vi "Preference_Panel.vi"(0 "Mode":T1) -> ()   [LabVIEW 2010]
uses:
  Anemometry Sub Vis/Controls/Server_Comms.ctl
  Anemometry Sub Vis/Controls/Preference_Mode.ctl
  Anemometry Sub Vis/File/Setup_Filetype.ctl
  Anemometry Sub Vis/Controls/Overhead.ctl
  <vilib>/Instr/_visa.llb/VISA Find Search Mode.ctl
  ADAM Client/Sub VIs/ADAM Controls/Calib_type_ADAM.ctl
  ADAM Client/Sub VIs/ADAM Controls/Module_type_ADAM.ctl
  ADAM Client/Sub VIs/ADAM Controls/Ch_description_ADAM.ctl
  ADAM Client/Sub VIs/ADAM Controls/Function_ADAM.ctl
  ADAM Client/Sub VIs/ADAM Controls/Channel_State.ctl
  ADAM Client/Sub VIs/ADAM Controls/Address.ctl
  Anemometry Sub Vis/Globals/Constants_global.vi
  Anemometry Sub Vis/Globals/Preference_global.vi
  Anemometry Sub Vis/Globals/Trav_pos_global.vi
  Anemometry Sub Vis/Globals/Qnet_Globals.vi
  Anemometry Sub Vis/Acquisition/PWA/PWAtasksGLOBAL.vi
  Anemometry Sub Vis/Globals/Dynamic_call_global.ph.vi
panel:
  in  "Post Processing Machine":bool
  in  "Analogue Device Serial No.":string="1188AB4"
  in  "PWA Device Serial No.":string="1187C98"
  in  "ADAM Setup File":u16(ring) items=["Scani_Valve.xls", "Current_Setup.xls"]
  in  "Default Source Establishment Time (s)":dbl=20.0
  out "This Machine's IP Number":string
  in  "Rig Setup":u16(ring) items=["3_x_2_tunnel", "A_Tunnel", "Adam_Sayer_Desk", "ADAM_Server", "Aero_Tunnel", "Alex_Desktop", "B_Tunnel", "Calibration_Tunnel", "Contact_Conductance", "D_Tunnel", "EnFlo_Tunnel", "Frauke_Desktop", "Fruit_Rig", "iMac_G5_2", "iMacDuo1", "Matteo's_desktop", "Matteo_PC", "Nick_PC-2", "Paul_Desk-Paul_Desk_Machine", "Paul_Hayden-Desk", "Paul_N_Desk_Machine_2", "phtest", "Post_Processing_Machine", "PowerBook_G4_1", "PowerBook_G4_2", "Syn_jet_rig", "Tank", "tdf", "Tom_Desk", "Towing_tank", "--New Rig Setup--"]
  in  "Default Traverse Name":u16(ring) items=["A_Tunnel", "Aero_Laser", "Aero_ThroughWall", "Aero_Tunnel", "Angle_Calibrator", "B_Tunnel", "D_Tunnel", "Dummy_Traverse", "EnFlo_Stack", "EnFlo_Tunnel", "EnFlo_Turntable", "Laser_Meas_Traverse", "mohd_setup", "Paul_Desk_Test", "PIV_Traverse", "--New Traverse Setup--"]
  in  "OK":bool
  in  "% Error From First Calib":dbl=10.0 format="%.1f"
  in  "% Error From Previous Calib":dbl=0.5 format="%.1f"
  in  "Qnet Site Root":path=path "/G4_2_HD/Users/paulhayden/Qnet/qnet"
  out "Templates":path=path "/G4_2_HD/Applications (Mac OS 9)/EnFlo Software/Anemometry/Anemometry Sub Vis/Templates"
  in  "Data Folder":path
  out "EnFlo SW Preferences":path=path "/G4_2_HD/Applications (Mac OS 9)/LabVIEW 5.1/EnFlo SW Preferences"
  in  "Tunnel Speed Control":bool
  in  "SMTP server IP address":string
  in  "Abs Press (mbar)":string="Froude:NPL:Atmos_Press"
  in  "Temperature":string="EnFlo Tun:Inlet Heater:Av Temp"
  in  "Server port number":u32=3363
  in  "Server address":string
  in  "LabVIEW Administrators":string[](array[string])=["", "", "", "", "", "", "", "", "", "", "", "", "", "", "", "", "", "", "", ""]
  in  "Server Comms":T2=enum."Do Not Link To Server"
  # "Server Computer Peferences"
  # "Multi Run Preferences"
  # "Warning Levels for Autocalibration Changes"
  # "Email Peferences"
  # "Deg C"
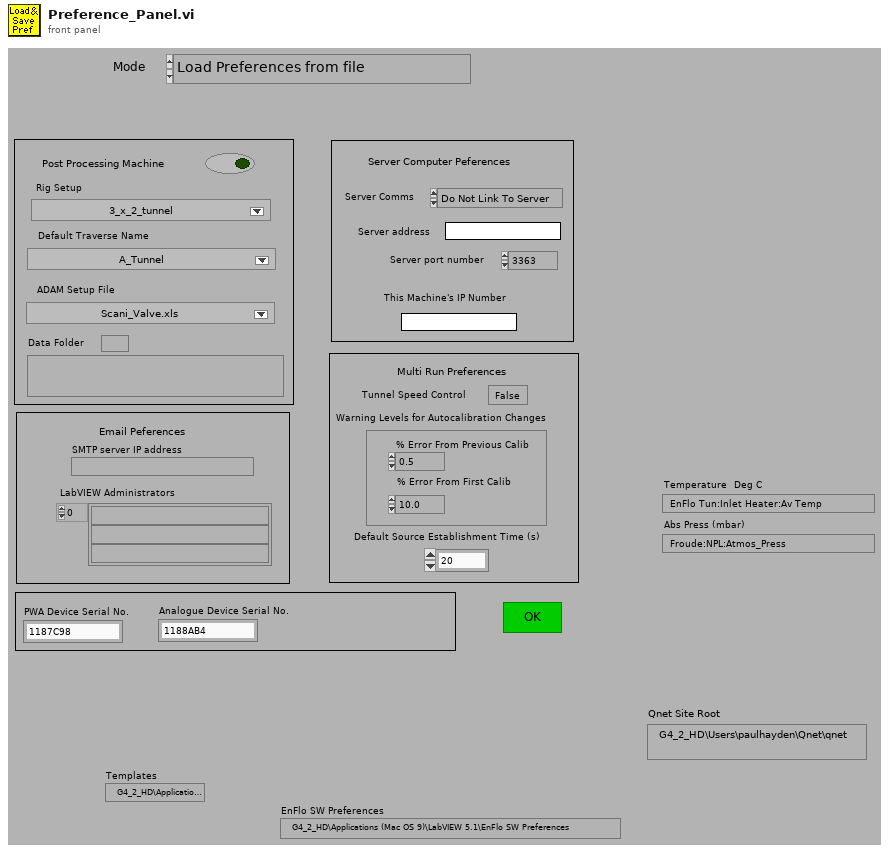
[diagram p1: front panel]
types:
  T1 = typedef "Preference_Mode.ctl" = enum16{"Load Preferences from file", "Save Preferences to file", "Load, Edit then Save"}
  T2 = typedef "Server_Comms.ctl" = enum16{"Server Link Healthy", "Do Not Link To Server"}
  T3 = enum8{"Enabled", "Disabled", "Disabled and Grayed Out"}
  T4 = typedef "Setup_Filetype.ctl" = enum16{"Measurement Setups", "Calibration Setups", "General", "Results File Plotter Setups", "Speed Calib Tweaks"}
  T5 = typedef "Overhead.ctl" = enum16{"Update total times", "Read Current Overhead", "Re Scale totals to 3 hrs", "Initialise totals to 3hr"}
  T6 = typedef "Calib_type_ADAM.ctl" = enum16{"Raw", "Bx + A", "Cx^2 + Bx + A", "Dx^3 + Cx^2 + Bx + A", "In Band", "Hi-Tec Q", "Hi-Tec M_dot", "Text"}
  T7 = typedef "Module_type_ADAM.ctl" = enum16{"4011", "4012", "4013", "4014", "4016", "4017", "4018", "4021", "4050", "4052", "4053", "4060", "4080", "5000", "5017", "5018", "5024", "5051", "5056", "5060", "6060", "Tracker", "WEST", "GILL", "JEM", "VICI", "Vaisala", "DRUCK", "Run VI Named:", "IR2100", "PPT", "Comparator", "VIRTUAL", "Hold Value", "Read A", "Read Ch", "Coded", "Client Info", "Web Client", "X10", "Test"}
  T8 = typedef "Channel_State.ctl" = enum16{"On", "Off", "Always On", "Always Off"}
  T9 = typedef "VISA Find Search Mode.ctl" = u32
  T10 = typedef "Ch_description_ADAM.ctl" = cluster{"Ch Name":string, "Type":T7, "Function":T11, "Ch State":T8, "Calibration type":T6, "A":dbl, "B":dbl, "C":dbl, "D":dbl, "Comments":string, "Address":T12, "String":string, "Duty":u16}
  T11 = typedef "Function_ADAM.ctl" = enum16{"Analogue Input", "Digital Input", "Event counter", "Event rate", "Analogue Output", "Digital Output", "Relay Output"}
  T12 = typedef "Address.ctl" = cluster{"Main":i32, "Ch.":i32, "Sub":i32, "Port Name":string}
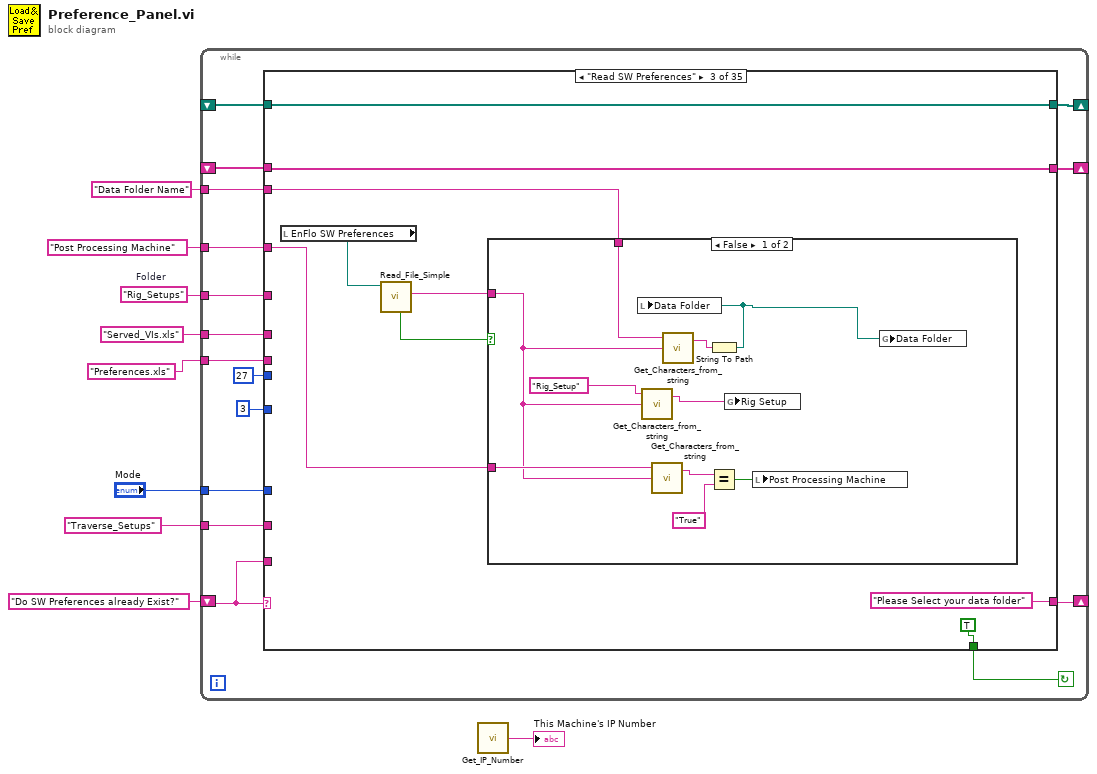
[diagram p0: block diagram]
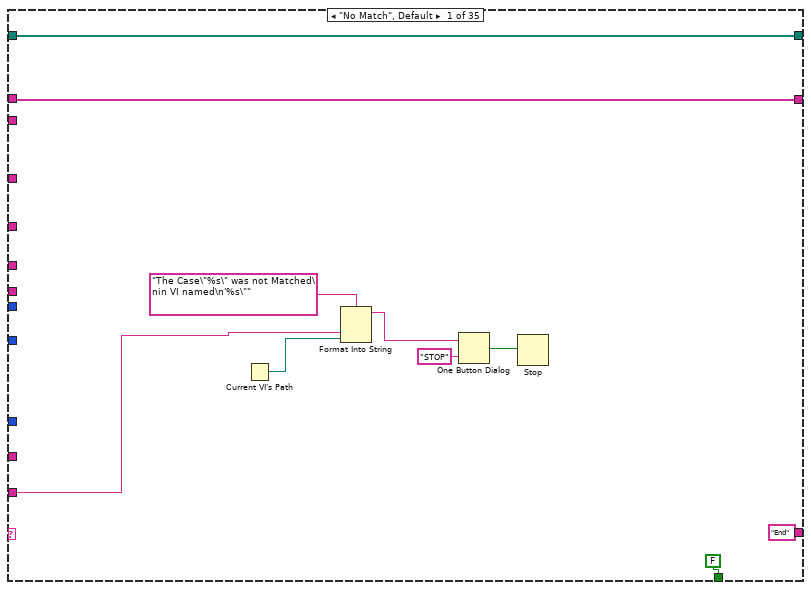
[diagram p2: hidden frame]
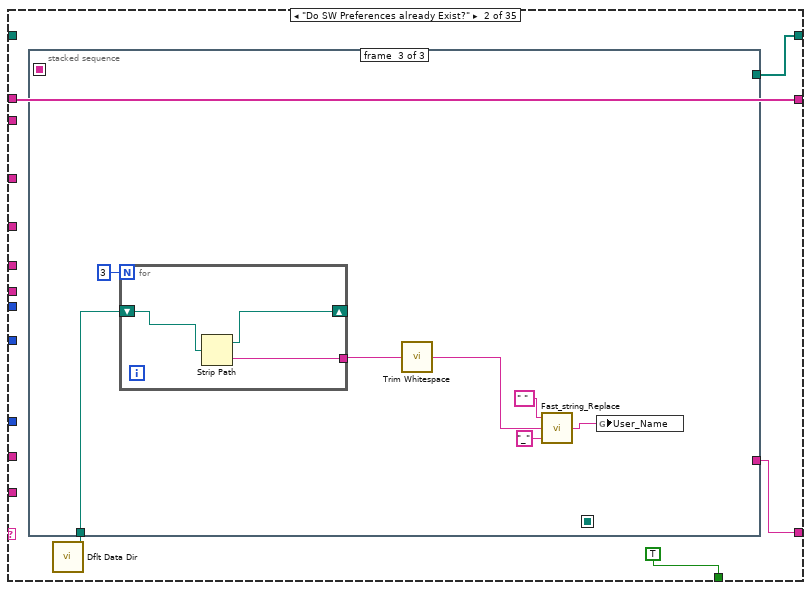
[diagram p3: hidden frame]
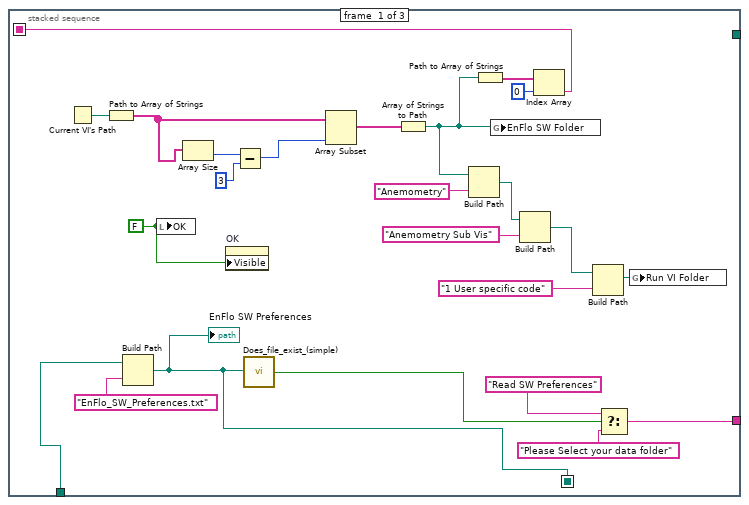
[diagram p4: hidden frame]
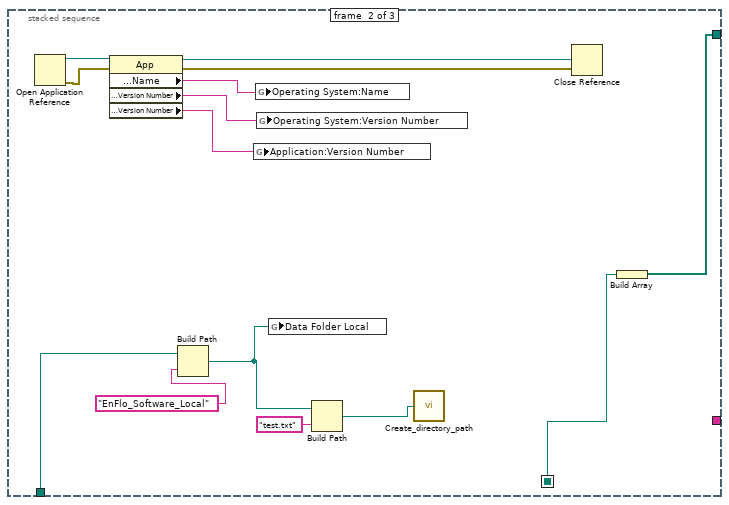
[diagram p5: hidden frame]
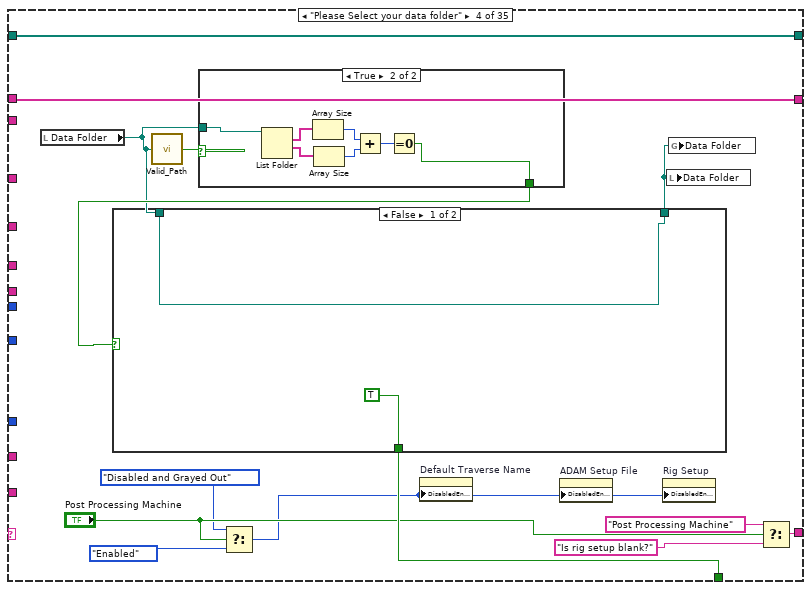
[diagram p7: hidden frame]
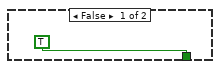
[diagram p8: hidden frame]
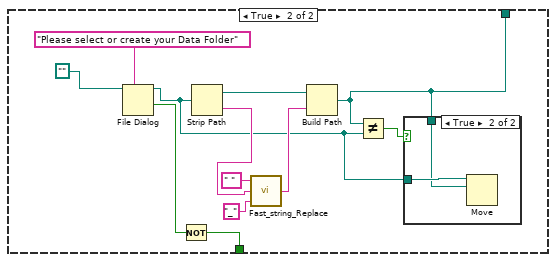
[diagram p9: hidden frame]
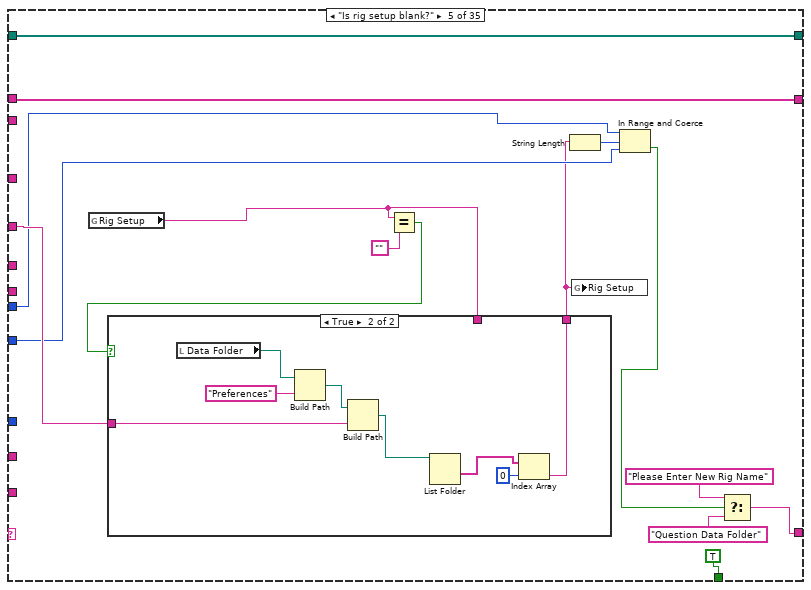
[diagram p11: hidden frame]
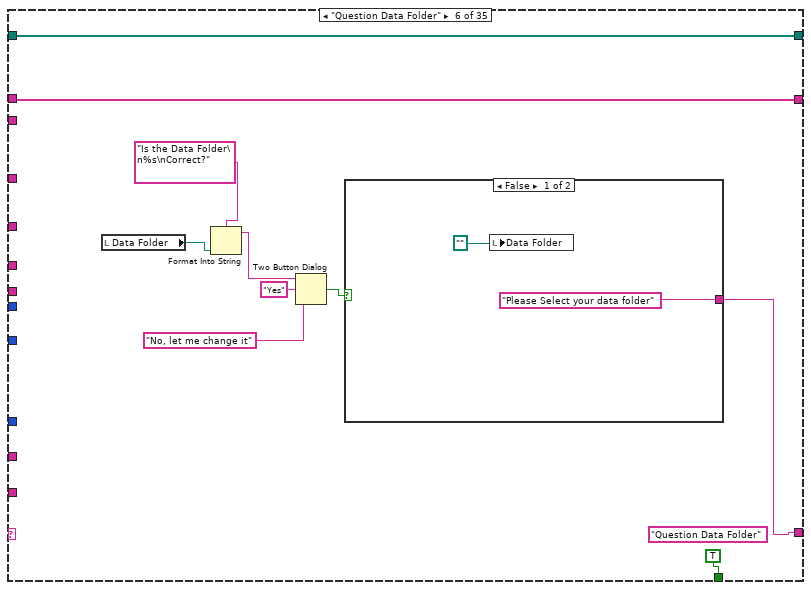
[diagram p13: hidden frame]
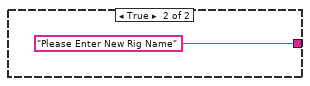
[diagram p14: hidden frame]
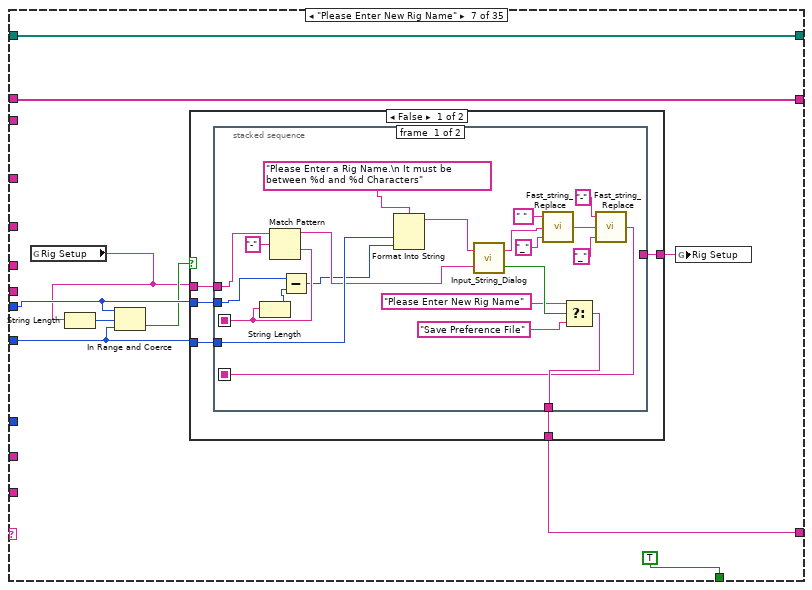
[diagram p15: hidden frame]
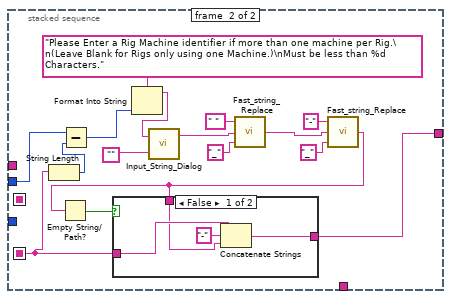
[diagram p16: hidden frame]
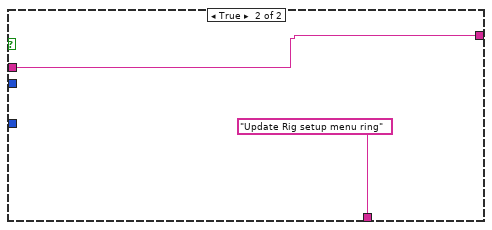
[diagram p18: hidden frame]
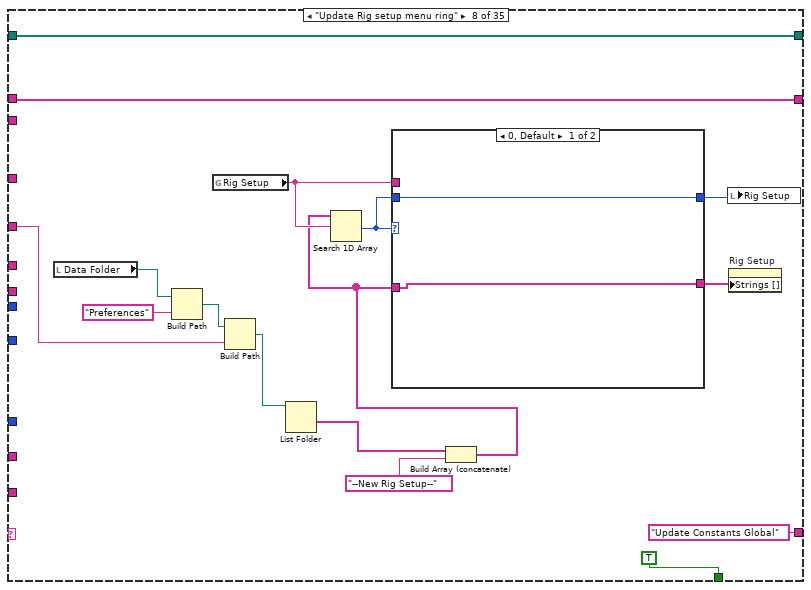
[diagram p19: hidden frame]
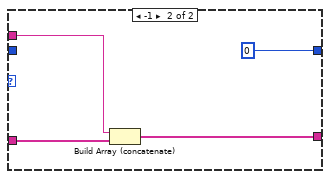
[diagram p20: hidden frame]
diagram:
  w4 = "Rig_Setups"  # Folder
  n1 = while {
    shift-left: _ -> [w22]
    shift-right: [w23] -> _
    shift-left: "Do SW Preferences already Exist?" -> [w21]
    shift-right: [w24] -> _
    tunnel: "Mode" -> [w20]
    tunnel: "Data Folder Name" ("Label for characters") -> [w19]
    tunnel: "Served_VIs.xls" ("Substring") -> [w18]
    tunnel: "Preferences.xls" ("name or relative path") -> [w17]
    tunnel: w4 -> [w14]
    tunnel: "Traverse_Setups" ("name or relative path") -> [w13]
    shift-right: [w12] -> _
    shift-left: _ -> [w11]
    tunnel: "Post Processing Machine" ("Label for characters") -> [w10]
    stop <- w25 continue-if-true
    n2 = case shown="\"Read SW Preferences\"" w21 {
      tunnel: [FALSE TRUE TRUE w115 TRUE TRUE TRUE TRUE TRUE TRUE TRUE TRUE TRUE TRUE TRUE TRUE TRUE TRUE TRUE TRUE TRUE TRUE TRUE TRUE TRUE TRUE TRUE TRUE TRUE TRUE w848 TRUE TRUE TRUE FALSE] -> w25
      tunnel: ["End" w38 "Please Select your data folder" w112 w147 w170 w189 "Update Constants Global" ("f") "Copy Preferences?" "Copy Preferences?" w316 "Read SW Preferences" "Install Preference files" "Install Adam table files" "Install Adam setup files" "Choose ADAM Setup file" "Preference files continued" "Variable Names" w487 w507 "Please Enter new  Traverse Setup" w579 "Create Traverse setup" ("f") "Check file permission status" w675 w704 w724 w743 w760 "Save Preference File" "Save SW Preferences" w912 w925 "Initialise Globals" "End"] -> w24
      tunnel: [w27 w39 w96 w121 w159 w178 w191 w256 w282 w304 w314 w328 w375 w390 w415 w434 w456 w466 w492 w514 w567 w581 w615 w632 w676 w709 w729 w752 w765 w779 w854 w920 w926 w978 w1038] -> w23
      tunnel: w22 -> [w27 w39 w96 w121 w159 w178 w191 w256 w282 w304 w314 w328 w375 w390 w415 w434 w456 w466 _ w514 w567 w581 w615 w632 w676 w709 w729 w752 w765 w779 w854 w920 w926 w978 w1038]
      tunnel: w21 -> [w30 _ _ _ _ _ _ _ _ _ _ _ _ _ _ _ _ _ _ _ _ _ _ _ _ _ _ _ _ _ _ _ _ _ _]
      tunnel: w20 -> [_ _ _ _ _ _ _ _ _ _ _ _ _ _ _ _ _ _ w486 _ _ _ _ _ w674 _ _ _ _ _ w849 _ _ _ _]
      tunnel: w19 -> [_ _ w93 _ _ _ _ _ _ _ _ _ _ _ _ _ _ _ _ _ _ _ _ _ _ _ _ _ _ _ _ w911 _ _ _]
      tunnel: w18 -> [_ _ _ _ _ _ _ _ _ _ _ _ _ w385 _ _ _ _ _ _ _ _ _ _ _ _ _ _ _ _ _ _ _ w970 _]
      tunnel: w17 -> [_ _ _ _ _ _ _ _ _ _ w310 w326 _ _ _ _ _ _ _ w504 _ _ _ _ _ _ _ _ _ _ w845 _ _ _ _]
      tunnel: 3 ("lower limit") -> [_ _ _ _ w151 _ w188 _ _ _ _ _ _ _ _ _ _ _ _ _ _ w578 _ _ _ _ _ _ _ _ _ _ _ _ _]
      tunnel: 27 ("upper limit") -> [_ _ _ _ w152 _ w187 _ _ _ _ _ _ _ _ _ _ _ _ _ _ w577 _ _ _ _ _ _ _ _ _ _ _ _ _]
      tunnel: w14 -> [_ _ _ _ w156 _ _ w244 w270 _ _ w325 _ _ _ _ _ _ _ _ _ _ _ _ _ _ _ _ _ _ _ _ _ _ _]
      tunnel: w13 -> [_ _ _ _ _ _ _ _ _ _ _ _ _ _ _ _ _ _ _ _ w565 _ w602 _ _ _ _ _ _ w778 _ _ _ _ _]
      tunnel: [w26 w36 w92 w116 w154 w177 w183 w242 w267 w293 w315 w329 w368 w381 w408 w431 w442 w458 w479 w510 w564 w573 w601 w628 path[] [] w701 w721 w746 w763 w777 w847 w908 w924 w972 w1035] -> w12
      tunnel: w11 -> [w26 _ w92 w116 w154 w177 w183 w242 w267 w293 w315 w329 w367 w383 w408 w432 w442 w460 w479 w511 w564 w573 w601 w629 w673 w701 w721 w746 w763 w777 w847 w908 w924 w972 w1035]
      tunnel: w10 -> [_ _ w91 _ _ _ _ _ _ _ _ _ _ _ _ _ _ _ _ _ _ _ _ _ _ _ _ _ _ _ _ w902 _ _ _]
      frame "No Match", Default {
        n3 = Current VI's Path() -> (path=w35:path)
        n4 = Format Into String(format string="The Case\"%s\" was not Matched\nin VI named\n'%s\"" ("Format String"), w30, w35) -> (resulting string=w32:string)  [unwired: 2 in, 1 out]
        n5 = One Button Dialog(message=w32, button name ("OK")="STOP") -> (true=w34:bool)
        n6 = Stop(stop? (T)=w34) -> ()
      }
      frame "Do SW Preferences already Exist?" {
        n7 = call <vilib>:"Dflt Data Dir.vi"() -> ("App:Default Data Directory"=w37:path)
        n8 = stacked-sequence {
          seq-local: [w44 _ _] -> [_ _ _]
          seq-local: [w42 _ _] -> [_ w70 _]
          tunnel: [w48 _ _] -> w38
          tunnel: w37 -> [w43 w68 w84]
          tunnel: [_ w71 _] -> w36
          frame #0 {
            w41 = FALSE ("OK")
            n9 = Current VI's Path() -> (path=w62:path)
            n10 = Path to Array of Strings(0:w62) -> (2:w59:string[])  [unwired: 1 out]
            n11 = Build Path(base path=w43, name or relative path="EnFlo_SW_Preferences.txt") -> (appended path=w42:path)
            "EnFlo SW Preferences" <- w42
            n12 = local write "OK"(w41) -> ()
            n13 = Array Size(array=w59) -> (size(s)=w61:i32)
            n14 = property on="OK" class="Bool (strict)"("Visible"=w41) -> ()  [unwired: 2 in, 2 out]
            n15 = Subtract(x=w61, y=3) -> (x-y=w57:i32)
            n16 = call "Does_file_exist_(simple).vi"("Pathname"=w42) -> ("exists?"=w63:bool)
            n17 = Array Subset(array=w59, length=w57) -> (w58:string[])  [unwired: 1 in]
            n18 = Array of Strings to Path(0:w58) -> (2:w45:path)  [unwired: 1 out]
            n19 = Build Path(base path=w45, name or relative path="Anemometry") -> (appended path=w54:path)
            n20 = Path to Array of Strings(0:w45) -> (2:w46:string[])  [unwired: 1 out]
            n21 = global write "Constants_global.vi" "EnFlo SW Folder"(w45) -> ()
            n22 = Build Path(base path=w54, name or relative path="Anemometry Sub Vis") -> (appended path=w52:path)
            n23 = Index Array(array=w46, index=0) -> (element=w44:string)
            n24 = Build Path(base path=w52, name or relative path="1 User specific code") -> (appended path=w51:path)
            n25 = Select(t="Read SW Preferences", s=w63, f="Please Select your data folder") -> (s? t:f=w48:string)
            n26 = global write "Constants_global.vi" "Run VI Folder"(w51) -> ()
          }
          frame #1 {
            n27 = Open Application Reference() -> (0:w75:errorcluster, 3:w78:refnum<vi>)  [unwired: 1 in, 3 out]
            n28 = property class="App"(reference=w78, error in=w75) -> (reference out=w77:refnum<vi>, error out=w76:errorcluster, "Operating System:Name"=w72:string, "Operating System:Version Number"=w74:string, "Application:Version Number"=w73:string)
            n29 = Build Path(base path=w68, name or relative path="EnFlo_Software_Local" ("element")) -> (appended path=w67:path)
            n30 = global write "Preference_global.vi" "Application:Version Number"(w73) -> ()
            n31 = global write "Preference_global.vi" "Operating System:Name"(w72) -> ()
            n32 = global write "Preference_global.vi" "Operating System:Version Number"(w74) -> ()
            n33 = global write "Constants_global.vi" "Data Folder Local"(w67) -> ()
            n34 = Build Path(base path=w67, name or relative path="test.txt") -> (appended path=w65:path)
            n35 = call "Create_directory_path.vi"("Path name"=w65) -> ()  [unwired: 1 out]
            n36 = Close Reference(reference=w77, error in (no error)=w76) -> ()  [unwired: 1 out]
            n37 = Build Array(w70) -> (w71:path[])
          }
          frame #2 {
            n38 = for {
              N: 3 -> [_]
              shift-right: [w88] -> _
              shift-left: w84 -> [w87]
              tunnel: [w86] -> w80
              n39 = Strip Path(path=w87) -> (stripped path=w88:path, name=w86:string)
            }
            n40 = call <vilib>:"Trim Whitespace.vi"("string"=w80) -> ("trimmed string"=w79:string)  [unwired: 1 in]
            n41 = call "Fast_string_Replace.vi"("Replace match with:"="_", "Input String"=w79, "regular expression"=" ") -> ("Output String"=w81:string)  [unwired: 1 in, 1 out]
            n42 = global write "Preference_global.vi" "User_Name"(w81) -> ()
          }
        }
      }
      frame "Read SW Preferences" {
        n43 = local read "EnFlo SW Preferences"() -> (w95:path)
        n44 = call "Read_File_Simple.vi"("Filename"=w95) -> ("Error?"=w89:bool, "string"=w90:string)  [unwired: 2 in, 6 out]
        n45 = case shown="False" w89 {
          tunnel: w93 -> [w106 _]
          tunnel: w91 -> [w102 _]
          tunnel: w90 -> [w101 _]
          frame False {
            n46 = call "Get_Characters_from_string.vi"("Input string"=w101, "Variable name"="Rig_Setup" ("Label for characters")) -> ("Value"=w103:string)  [unwired: 1 in, 1 out]
            n47 = call "Get_Characters_from_string.vi"("Input string"=w101, "Variable name"=w102) -> ("Value"=w100:string)  [unwired: 1 in, 1 out]
            n48 = call "Get_Characters_from_string.vi"("Input string"=w101, "Variable name"=w106) -> ("Value"=w107:string)  [unwired: 1 in, 1 out]
            n49 = String To Path(string=w107) -> (path=w105:path)
            n50 = local write "Data Folder"(w105) -> ()
            n51 = Equal?(x=w100, y="True") -> (x = y?=w98:bool)
            n52 = global write "Preference_global.vi" "Rig Setup"(w103) -> ()
            n53 = local write "Post Processing Machine"(w98) -> ()
            n54 = global write "Constants_global.vi" "Data Folder"(w105) -> ()
          }
          frame True {
          }
        }
      }
      frame "Please Select your data folder" {
        n55 = local read "Data Folder"() -> (w117:path)
        n56 = call "Valid_Path.vi"("Filename"=w117) -> ("Valid Path?"=w119:bool)
        n57 = case shown="True" w119 {
          tunnel: [TRUE ("status") w123] -> w118
          tunnel: w117 -> [_ w129]
          frame False {
          }
          frame True {
            n58 = List Folder(path=w129) -> (filenames=w127:string[], folder names=w128:string[])  [unwired: 1 in, 4 out]
            n59 = Array Size(array=w127) -> (size(s)=w125:i32)
            n60 = Array Size(array=w128) -> (size(s)=w126:i32)
            n61 = Add(x=w125, y=w126) -> (x+y=w124:i32)
            n62 = Equal To 0?(x=w124) -> (x = 0?=w123:bool)
          }
        }
        n63 = case shown="False" w118 {
          tunnel: [w131 w134] -> w120
          tunnel: w117 -> [w131 _]
          tunnel: [TRUE w132] -> w115
          frame False {
          }
          frame True {
            n64 = File Dialog(7:"Please select or create your Data Folder" ("prompt"), 11:path "") -> (1:w133:bool, 3:w135:path)  [unwired: 1 in, 6 out]
            n65 = Not(x=w133) -> (.not. x?=w132:bool)
            n66 = Strip Path(path=w135) -> (stripped path=w139:path, name=w138:string)
            n67 = call "Fast_string_Replace.vi"("Replace match with:"="_", "Input String"=w138, "regular expression"=" ") -> ("Output String"=w137:string)  [unwired: 2 out]
            n68 = Build Path(base path=w139, name or relative path=w137) -> (appended path=w134:path)
            n69 = Not Equal?(x=w134, y=w135) -> (x != y?=w136:bool)
            n70 = case shown="True" w136 {
              tunnel: w135 -> [_ w145]
              tunnel: w134 -> [_ w144]
              frame False {
              }
              frame True {
                n71 = Move(source path=w145, 10:w144) -> ()  [unwired: 1 in, 5 out]
              }
            }
          }
        }
        n72 = Select(t=T3."Disabled and Grayed Out" ("Disabled"), s="Post Processing Machine", f=T3."Enabled" ("Disabled")) -> (s? t:f=w108:T3)
        n73 = property on="Default Traverse Name" class="Ring (strict)"("DisabledEnum"=w108) -> ()  [unwired: 2 in, 2 out]
        n74 = property on="ADAM Setup File" class="Ring (strict)"("DisabledEnum"=w108) -> ()  [unwired: 2 in, 2 out]
        n75 = property on="Rig Setup" class="Ring (strict)"("DisabledEnum"=w108) -> ()  [unwired: 2 in, 2 out]
        n76 = local write "Data Folder"(w120) -> ()
        n77 = global write "Constants_global.vi" "Data Folder"(w120) -> ()
        n78 = Select(t="Post Processing Machine", s="Post Processing Machine", f="Is rig setup blank?") -> (s? t:f=w112:string)
      }
      frame "Is rig setup blank?" {
        n79 = global read "Preference_global.vi" "Rig Setup"() -> (w155:string)
        n80 = Equal?(x=w155, y="") -> (x = y?=w157:bool)
        n81 = case shown="True" w157 {
          tunnel: w156 -> [_ w165]
          tunnel: [w161 w162] -> w150
          tunnel: w155 -> [w161 _]
          frame False {
          }
          frame True {
            n82 = local read "Data Folder"() -> (w168:path)
            n83 = Build Path(base path=w168, name or relative path="Preferences") -> (appended path=w167:path)
            n84 = Build Path(base path=w167, name or relative path=w165) -> (appended path=w166:path)
            n85 = List Folder(path=w166) -> (folder names=w163:string[])  [unwired: 1 in, 5 out]
            n86 = Index Array(array=w163, index=0) -> (element=w162:string)
          }
        }
        n87 = String Length(string=w150) -> (length=w153:i32)
        n88 = global write "Preference_global.vi" "Rig Setup"(w150) -> ()
        n89 = In Range and Coerce(upper limit=w152, x=w153, lower limit=w151) -> (In Range?=w149:bool)  [unwired: 1 out]
        n90 = Select(t="Please Enter New Rig Name", s=w149, f="Question Data Folder") -> (s? t:f=w147:string)
      }
      frame "Question Data Folder" {
        (unwired) "Question Data Folder"
        n91 = local read "Data Folder"() -> (w176:path)
        n92 = Format Into String(format string="Is the Data Folder\n%s\nCorrect?" ("message"), w176) -> (resulting string=w174:string)  [unwired: 2 in, 1 out]
        n93 = Two Button Dialog(message=w174, 1:"No, let me change it" ("F button name (\"Cancel\")"), 2:"Yes" ("T button name (\"OK\")")) -> (T button?=w171:bool)
        n94 = case shown="False" w171 {
          tunnel: ["Please Select your data folder" "Please Enter New Rig Name"] -> w170
          frame False {
            n95 = local write "Data Folder"(path "") -> ()
          }
          frame True {
          }
        }
      }
      frame "Please Enter New Rig Name" {
        n96 = global read "Preference_global.vi" "Rig Setup"() -> (w185:string)
        n97 = String Length(string=w185) -> (length=w190:i32)
        n98 = In Range and Coerce(upper limit=w187, x=w190, lower limit=w188) -> (In Range?=w186:bool)  [unwired: 1 out]
        n99 = case shown="False" w186 {
          tunnel: w185 -> [w197 w240]
          tunnel: [w193 "Update Rig setup menu ring"] -> w189
          tunnel: [w194 w240] -> w184
          tunnel: w188 -> [w196 _]
          tunnel: w187 -> [w195 _]
          frame False {
            n100 = stacked-sequence {
              seq-local: [w198 _] -> [_ w223]
              seq-local: [w205 _] -> [_ _]
              tunnel: w197 -> [w207 _]
              tunnel: w196 -> [w218 _]
              tunnel: w195 -> [w204 w221]
              tunnel: [_ w226] -> w194
              tunnel: [w210 _] -> w193
              frame #0 {
                n101 = Match Pattern(string=w207, regular expression="-") -> (before substring=w206:string, after substring=w205:string)  [unwired: 3 out]
                n102 = String Length(string=w205) -> (length=w203:i32)
                n103 = Subtract(x=w204, y=w203) -> (x-y=w202:i32)
                n104 = Format Into String(format string="Please Enter a Rig Name.\n It must be between %d and %d Characters" ("Message to user"), w218, w202) -> (resulting string=w217:string)  [unwired: 2 in, 1 out]
                n105 = call "Input_String_Dialog.vi"("Value"=w206, "Message to user"=w217) -> ("Ok Out"=w213:bool, "Output string"=w214:string)
                n106 = call "Fast_string_Replace.vi"("Replace match with:"="_", "Input String"=w214, "regular expression"=" ") -> ("Output String"=w199:string)  [unwired: 2 out]
                n107 = Select(t="Please Enter New Rig Name", s=w213, f="Save Preference File") -> (s? t:f=w210:string)
                n108 = call "Fast_string_Replace.vi"("Replace match with:"="_", "Input String"=w199, "regular expression"="-") -> ("Output String"=w198:string)  [unwired: 2 out]
              }
              frame #1 {
                n109 = String Length(string=w223) -> (length=w222:i32)
                n110 = Subtract(x=w221, y=w222) -> (x-y=w220:i32)
                n111 = Format Into String(format string="Please Enter a Rig Machine identifier if more than one machine per Rig.\n(Leave Blank for Rigs only using one Machine.)\nMust be less than %d Characters." ("Message to user"), w220) -> (resulting string=w219:string)  [unwired: 2 in, 1 out]
                n112 = call "Input_String_Dialog.vi"("Value"="", "Message to user"=w219) -> ("Output string"=w232:string)  [unwired: 1 out]
                n113 = call "Fast_string_Replace.vi"("Replace match with:"="_", "Input String"=w232, "regular expression"=" ") -> ("Output String"=w228:string)  [unwired: 2 out]
                n114 = call "Fast_string_Replace.vi"("Replace match with:"="_", "Input String"=w228, "regular expression"="-") -> ("Output String"=w225:string)  [unwired: 2 out]
                n115 = Empty String/Path?(string/path=w225) -> (empty?=w227:bool)
                n116 = case shown="False" w227 {
                  tunnel: [w235 w239] -> w226
                  tunnel: w223 -> [w238 w239]
                  tunnel: w225 -> [w236 _]
                  frame False {
                    n117 = Concatenate Strings(w238, "-" ("string"), w236) -> (w235:string)
                  }
                  frame True {
                  }
                }
              }
            }
          }
          frame True {
          }
        }
        n118 = global write "Preference_global.vi" "Rig Setup"(w184) -> ()
      }
      frame "Update Rig setup menu ring" {
        n119 = local read "Data Folder"() -> (w247:path)
        n120 = Build Path(base path=w247, name or relative path="Preferences") -> (appended path=w246:path)
        n121 = global read "Preference_global.vi" "Rig Setup"() -> (w253:string)
        n122 = Build Path(base path=w246, name or relative path=w244) -> (appended path=w245:path)
        n123 = List Folder(path=w245) -> (folder names=w243:string[])  [unwired: 1 in, 5 out]
        n124 = Build Array (concatenate)(w243, "--New Rig Setup--") -> (w249:string[])
        n125 = Search 1D Array(1D array=w249, element=w253) -> (index of element=w252:i32)  [unwired: 1 out]
        n126 = case shown="0, Default" w252 {
          tunnel: [w259 0] -> w255
          tunnel: w249 -> [w258 w262]
          tunnel: w253 -> [_ w261]
          tunnel: w252 -> [w259 _]
          tunnel: [w258 w260] -> w251
          frame 0, Default {
          }
          frame -1 {
            n127 = Build Array (concatenate)(w261, w262) -> (w260:string[])
          }
        }
        n128 = local write "Rig Setup"(w255) -> ()
        n129 = property on="Rig Setup" class="Ring (strict)"("Strings []"=w251) -> ()  [unwired: 2 in, 2 out]
      }
      frame "Update Constants Global" {
        n130 = global read "Constants_global.vi" "Data Folder"() -> (w268:path)
        n131 = global read "Preference_global.vi" "Rig Setup"() -> (w269:string)
        n132 = Build Path(base path=w268, name or relative path="Preferences") -> (appended path=w271:path)
        n133 = Build Path(base path=w271, name or relative path=w270) -> (appended path=w272:path)
        n134 = Build Path(base path=w272, name or relative path=w269) -> (appended path=w264:path)
        n135 = Build Path(base path=w264, name or relative path="ADAM table") -> (appended path=w277:path)
        n136 = Build Path(base path=w264, name or relative path="Serial") -> (appended path=w276:path)
        n137 = Build Path(base path=w264, name or relative path="All_Users") -> (appended path=w265:path)
        n138 = Build Path(base path=w271, name or relative path="Traverse_Setups") -> (appended path=w275:path)
        n139 = global write "Constants_global.vi" "ADAM setups folder"(w277) -> ()
        n140 = global write "Constants_global.vi" "Serial setups folder"(w276) -> ()
        n141 = global write "Constants_global.vi" "All_Users"(w265) -> ()
        n142 = global write "Constants_global.vi" "Traverse folder"(w275) -> ()
        n143 = Build Array(w277, w276, w265, w275) -> (w274:path[])
        n144 = for {
          tunnel: w274 -> [w286] mode=indexing
          n145 = Build Path(base path=w286, name or relative path="Test") -> (appended path=w284:path)
          n146 = call "Create_directory_path.vi"("Path name"=w284) -> ()  [unwired: 1 out]
        }
      }
      frame "Post Processing Machine" {
        n147 = global read "Constants_global.vi" "Data Folder Local"() -> (w292:path)
        n148 = global read "Preference_global.vi" "User_Name"() -> (w287:string)
        n149 = Build Path(base path=w292, name or relative path="Preferences") -> (appended path=w294:path)
        n150 = Build Path(base path=w294, name or relative path=w287) -> (appended path=w288:path)
        n151 = Build Path(base path=w288, name or relative path="ADAM table") -> (appended path=w299:path)
        n152 = Build Path(base path=w288, name or relative path="Serial") -> (appended path=w298:path)
        n153 = Build Path(base path=w288, name or relative path="All_Users") -> (appended path=w289:path)
        n154 = Build Path(base path=w294, name or relative path="Traverse_Setups") -> (appended path=w297:path)
        n155 = global write "Constants_global.vi" "ADAM setups folder"(w299) -> ()
        n156 = global write "Constants_global.vi" "Serial setups folder"(w298) -> ()
        n157 = global write "Constants_global.vi" "All_Users"(w289) -> ()
        n158 = global write "Constants_global.vi" "Traverse folder"(w297) -> ()
        n159 = Build Array(w299, w298, w289, w297) -> (w296:path[])
        n160 = for {
          tunnel: w296 -> [w308] mode=indexing
          n161 = Build Path(base path=w308, name or relative path="Test") -> (appended path=w306:path)
          n162 = call "Create_directory_path.vi"("Path name"=w306) -> ()  [unwired: 1 out]
        }
        n163 = global write "Preference_global.vi" "Rig Setup"("Post_Processing_Machine" ("Rig Setup")) -> ()
      }
      frame "Copy Preferences?" {
        n164 = call "Setup_Filepath.vi"("Setup File Type"=Setup_Filetype."General", "Filename in"=w310) -> ("Filename Out"=w309:path)  [unwired: 1 out]
        n165 = call <vilib>:"Check if File or Folder Exists.vi"("path"=w309) -> ("file or folder exists?"=w313:bool)  [unwired: 1 in, 9 out]
        n166 = case shown="False" w313 {
          tunnel: [w320 TRUE ("Error?")] -> w312
          frame False {
            n167 = global read "Constants_global.vi" "All_Users"() -> (w322:path)
            n168 = Build Path(base path=w322, name or relative path="Current_Username") -> (appended path=w323:path)
            n169 = call "Read_File_Simple.vi"("Filename"=w323) -> ("Error?"=w320:bool)  [unwired: 4 in, 5 out]
          }
          frame True {
          }
        }
        n170 = Select(t="Install Generic Meas Setup file", s=w312, f="Copy from last user") -> (s? t:f=w316:string)
      }
      frame "Copy from last user" {
        n171 = stacked-sequence {
          seq-local: [w335 _ _ _] -> [_ w346 w353 w360]
          tunnel: w326 -> [_ w344 _ _]
          tunnel: w325 -> [w331 _ _ _]
          frame #0 {
            n172 = global read "Constants_global.vi" "All_Users"() -> (w340:path)
            n173 = global read "Constants_global.vi" "Data Folder"() -> (w334:path)
            n174 = Build Path(base path=w340, name or relative path="Current_Username") -> (appended path=w338:path)
            n175 = global read "Preference_global.vi" "Rig Setup"() -> (w342:string)
            n176 = call "Read_File_Simple.vi"("Filename"=w338) -> ("string"=w337:string)  [unwired: 4 in, 5 out]
            n177 = Build Path(base path=w334, name or relative path="Preferences") -> (appended path=w333:path)
            n178 = Build Path(base path=w333, name or relative path=w331) -> (appended path=w332:path)
            n179 = Build Path(base path=w332, name or relative path=w342) -> (appended path=w336:path)
            n180 = Build Path(base path=w336, name or relative path=w337) -> (appended path=w335:path)
          }
          frame #1 {
            n181 = call "Setup_Filepath.vi"("Setup File Type"=Setup_Filetype."General", "Filename in"=w344) -> ("Filename Out"=w343:path)  [unwired: 1 out]
            n182 = Build Path(base path=w346, name or relative path="General") -> (appended path=w348:path)
            n183 = Build Path(base path=w348, name or relative path=w344) -> (appended path=w347:path)
            n184 = Copy(10:w343, 11:w347) -> ()  [unwired: 3 in, 3 out]
          }
          frame #2 {
            w351 = "Current_Setup.xls"
            n185 = Build Path(base path=w353, name or relative path="Meas Setups") -> (appended path=w355:path)
            n186 = Build Path(base path=w355, name or relative path=w351) -> (appended path=w354:path)
            n187 = call "Setup_Filepath.vi"("Setup File Type"=Setup_Filetype."Measurement Setups", "Filename in"=w351) -> ("Filename Out"=w350:path)  [unwired: 1 out]
            n188 = Copy(10:w350, 11:w354) -> ()  [unwired: 3 in, 3 out]
          }
          frame #3 {
            w358 = "Current_Setup.xls"
            n189 = Build Path(base path=w360, name or relative path="Calib Setups") -> (appended path=w362:path)
            n190 = Build Path(base path=w362, name or relative path=w358) -> (appended path=w361:path)
            n191 = call "Setup_Filepath.vi"("Setup File Type"=Setup_Filetype."Calibration Setups", "Filename in"=w358) -> ("Filename Out"=w357:path)  [unwired: 1 out]
            n192 = Copy(10:w357, 11:w361) -> ()  [unwired: 3 in, 3 out]
          }
        }
      }
      frame "Install Generic Meas Setup file" {
        n193 = global read "Constants_global.vi" "Run VI Folder"() -> (w374:path)
        n194 = Strip Path(path=w374) -> (stripped path=w372:path)  [unwired: 1 out]
        n195 = call "Setup_Filepath.vi"("Setup File Type"=Setup_Filetype."Measurement Setups", "Filename in"="Current_Setup.xls" ("name or relative path")) -> ("Filename Out"=w364:path)  [unwired: 1 out]
        n196 = Build Path(base path=w372, name or relative path="Templates") -> (appended path=w370:path)
        "Templates" <- w370
        n197 = call "Does_file_exist_(simple).vi"("Pathname"=w364) -> ("exists?"=w371:bool)
        n198 = case shown="False" w371 {
          tunnel: w364 -> [w380 _]
          tunnel: w370 -> [w378 _]
          frame False {
            n199 = Build Path(base path=w378, name or relative path="Measurement Setup.xls") -> (appended path=w377:path)
            n200 = Copy(10:w380, 11:w377) -> ()  [unwired: 1 in, 5 out]
          }
          frame True {
          }
        }
        n201 = Build Array (concatenate)(w367, w364) -> (w368:path[])
      }
      frame "Install Preference files" {
        n202 = Build Array("Preferences.xls" ("Substring"), w385, "Month_Names.xls" ("name or relative path"), "LDA_Configuration.xls") -> (w389:string[])
        n203 = for {
          tunnel: w389 -> [w393] mode=indexing
          tunnel: [w392] -> w382 mode=indexing
          n204 = call "Setup_Filepath.vi"("Setup File Type"=Setup_Filetype."General", "Filename in"=w393) -> ("Filename Out"=w392:path)  [unwired: 1 out]
          n205 = call "Does_file_exist_(simple).vi"("Pathname"=w392) -> ("exists?"=w395:bool)
          n206 = case shown="False" w395 {
            tunnel: w392 -> [w399 _]
            tunnel: w393 -> [w396 _]
            frame False {
              n207 = local read "Templates"() -> (w397:path)
              n208 = Build Path(base path=w397, name or relative path=w396) -> (appended path=w398:path)
              n209 = Copy(10:w399, 11:w398) -> ()  [unwired: 1 in, 5 out]
            }
            frame True {
            }
          }
        }
        n210 = Build Array (concatenate)(w383, w382) -> (w381:path[])
      }
      frame "Install Adam table files" {
        w404 = "Current_Setup.xls"
        n211 = global read "Constants_global.vi" "ADAM setups folder"() -> (w406:path)
        n212 = Build Path(base path=w406, name or relative path=w404) -> (appended path=w407:path)
        n213 = Build Path(base path=w406, name or relative path="Setup_Files") -> (appended path=w402:path)
        n214 = Build Array("Hi_Tec_Calibs.xls" ("name or relative path"), "A_Tunnel DB setup.xls" ("Substring"), "EnFlo_Tunnel DB setup.xls", "Aero_Tunnel DB setup.xls" ("name or relative path"), "D_Tunnel DB setup.xls") -> (w414:string[])
        n215 = Build Path(base path=w402, name or relative path=w404) -> (appended path=w401:path)
        n216 = for {
          tunnel: w414 -> [w418] mode=indexing
          tunnel: w406 -> [w419]
          n217 = Build Path(base path=w419, name or relative path=w418) -> (appended path=w417:path)
          n218 = call "Does_file_exist_(simple).vi"("Pathname"=w417) -> ("exists?"=w420:bool)
          n219 = case shown="False" w420 {
            tunnel: w417 -> [w424 _]
            tunnel: w418 -> [w421 _]
            frame False {
              n220 = local read "Templates"() -> (w422:path)
              n221 = Build Path(base path=w422, name or relative path=w421) -> (appended path=w423:path)
              n222 = Copy(10:w424, 11:w423) -> ()  [unwired: 1 in, 5 out]
            }
            frame True {
            }
          }
        }
        n223 = call "Create_directory_path.vi"("Path name"=w401) -> ("Path name Out"=w400:path)
        n224 = Move(source path=w407, 10:w400) -> ()  [unwired: 1 in, 5 out]
      }
      frame "Install Adam setup files" {
        w428 = "Current_Setup.xls"
        n225 = global read "Constants_global.vi" "ADAM setups folder"() -> (w430:path)
        n226 = Build Path(base path=w430, name or relative path="Setup_Files") -> (appended path=w427:path)
        n227 = Build Path(base path=w427, name or relative path=w428) -> (appended path=w425:path)
        n228 = call "Does_file_exist_(simple).vi"("Pathname"=w425) -> ("exists?"=w426:bool)
        n229 = case shown="False" w426 {
          tunnel: w425 -> [w441 _]
          tunnel: w428 -> [w439 _]
          frame False {
            n230 = local read "Templates"() -> (w440:path)
            n231 = Build Path(base path=w440, name or relative path="ADAM_Setup_files") -> (appended path=w438:path)
            n232 = Build Path(base path=w438, name or relative path=w439) -> (appended path=w437:path)
            n233 = Copy(10:w441, 11:w437) -> ()  [unwired: 1 in, 5 out]
          }
          frame True {
          }
        }
        n234 = Build Array (concatenate)(w432, w425) -> (w431:path[])
      }
      frame "Choose ADAM Setup file" {
        w450 = "Selected_Filename.txt" ("Substring")
        n235 = global read "Constants_global.vi" "ADAM setups folder"() -> (w454:path)
        n236 = Build Path(base path=w454, name or relative path="Setup_Files") -> (appended path=w451:path)
        n237 = Build Path(base path=w451, name or relative path=w450) -> (appended path=w449:path)
        n238 = call "Read_File_Simple.vi"("Filename"=w449) -> ("string"=w447:string)  [unwired: 2 in, 7 out]
        n239 = Build Array(w450) -> (w452:string[])
        n240 = call "List_files_in_order_of_age.vi"("Files to Hide"=w452, "Folder"=w451) -> ("file names"=w448:string[])
        n241 = Search 1D Array(1D array=w448, element=w447) -> (index of element=w444:i32)  [unwired: 1 out]
        n242 = property on="ADAM Setup File" class="Ring (strict)"("Strings []"=w448) -> ()  [unwired: 2 in, 2 out]
        n243 = Less Than 0?(x=w444) -> (x < 0?=w445:bool)
        n244 = Select(t=0, s=w445, f=w444) -> (s? t:f=w443:i32)
        n245 = local write "ADAM Setup File"(w443) -> ()
      }
      frame "Preference files continued" {
        n246 = Build Array("Hot_Wire_Bridges.txt", "Hot_Wire_Probes.txt", "Pressure_Transducers.txt") -> (w461:string[])
        n247 = for {
          tunnel: w461 -> [w469] mode=indexing
          tunnel: [w468] -> w459 mode=indexing
          n248 = call "Setup_Filepath.vi"("Setup File Type"=Setup_Filetype."Calibration Setups", "Filename in"=w469) -> ("Filename Out"=w468:path)  [unwired: 1 out]
          n249 = call "Does_file_exist_(simple).vi"("Pathname"=w468) -> ("exists?"=w471:bool)
          n250 = case shown="False" w471 {
            tunnel: w468 -> [w475 _]
            tunnel: w469 -> [w472 _]
            frame False {
              n251 = local read "Templates"() -> (w473:path)
              n252 = Build Path(base path=w473, name or relative path=w472) -> (appended path=w474:path)
              n253 = Copy(10:w475, 11:w474) -> ()  [unwired: 1 in, 5 out]
            }
            frame True {
            }
          }
        }
        n254 = Build Array (concatenate)(w460, w459) -> (w458:path[])
      }
      frame "Variable Names" {
        n255 = Build Array("PWA Device Serial No.", "Analogue Device Serial No.", "Server address", "Server port number", "LabVIEW Administrators", "SMTP server IP address", "Server Comms", "Default Source Establishment Time (s)", "Temperature", "Abs Press (mbar)", "Default Traverse Name", "Tunnel Speed Control", "Current Overhead Factor", "Qnet Site Root", "Auto Calib Error fr Previous", "Auto Calib Error fr First") -> (w492:string[])
        n256 = case shown="\"Load, Edit then Save\"" w486 {
          tunnel: ["Load From Preference file" w498 "Save Preference File"] -> w487
          frame "Load Preferences from file" {
          }
          frame "Load, Edit then Save" {
            n257 = local read "OK"() -> (w501:bool)
            n258 = Select(t="Save Preference File", s=w501, f="Load From Preference file") -> (s? t:f=w498:string)
          }
          frame "Save Preferences to file" {
          }
        }
      }
      frame "Load From Preference file" {
        n259 = call "Setup_Filepath.vi"("Setup File Type"=Setup_Filetype."General", "Filename in"=w504) -> ("Filename Out"=w503:path)  [unwired: 1 out]
        n260 = call "Read_File_Simple.vi"("Filename"=w503) -> ("string"=w512:string)  [unwired: 2 in, 7 out]
        n261 = for {
          tunnel: w514 -> [w517] mode=indexing
          tunnel: w512 -> [w516]
          w519 = FALSE  # Show Dialog?
          n262 = call "Get_Characters_from_string.vi"("Show Dialog?"=w519, "Input string"=w516, "Variable name"=w517) -> ("Status"=w518:enum16{"Char in string", "Char not in string"}, "Value"=w515:string)
          n263 = case shown="\"Char in string\"" w518 {
            tunnel: w517 -> [w521 _]
            tunnel: w515 -> [w520 _]
            frame "Char in string" {
              n264 = case shown="\"Server address\"" w521 {
                tunnel: w521 -> [w523 _ _ _ _ _ _ _ _ _ _ _ _ _ _ _ _]
                tunnel: w520 -> [_ w524 w525 w528 w529 w530 w532 w534 w537 _ w541 w545 w546 w548 w550 w553 w555]
                tunnel: w520 -> [_ _ _ _ _ _ _ _ _ w538 _ _ _ _ _ _ _]
                frame "No Match", Default {
                  n265 = call "Was_string_matched.vi"("Match Error"=TRUE, "Variable name"=w523) -> ()  [unwired: 1 in]
                }
                frame "Server address" {
                  n266 = global write "Preference_global.vi" "Server address"(w524) -> ()
                  n267 = local write "Server address"(w524) -> ()
                }
                frame "Default Traverse Name" {
                  n268 = global write "Trav_pos_global.vi" "Default Traverse Setup"(w525) -> ()
                }
                frame "Server port number" {
                  n269 = Decimal String To Number(string=w528) -> (number=w527:i32)  [unwired: 3 out]
                  n270 = To Unsigned Long Integer(number=w527) -> (unsigned 32bit integer=w526:u32)
                  n271 = local write "Server port number"(w526) -> ()
                  n272 = global write "Preference_global.vi" "Server port number"(w526) -> ()
                }
                frame "Analogue Device Serial No." {
                  n273 = local write "Analogue Device Serial No."(w529) -> ()
                }
                frame "PWA Device Serial No." {
                  n274 = local write "PWA Device Serial No."(w530) -> ()
                }
                frame "Default Source Establishment Time (s)" {
                  n275 = Fract/Exp String To Number(string=w532) -> (number=w531:dbl)  [unwired: 4 out]
                  n276 = global write "Preference_global.vi" "Default Source Establishment Time (s)"(w531) -> ()
                  n277 = local write "Default Source Establishment Time (s)"(w531) -> ()
                }
                frame "Tunnel Speed Control" {
                  n278 = Equal?(x="TRUE", y=w534) -> (x = y?=w533:bool)
                  n279 = local write "Tunnel Speed Control"(w533) -> ()
                  n280 = global write "Preference_global.vi" "Tunnel Speed Control"(w533) -> ()
                }
                frame "LabVIEW Administrators" {
                  n281 = call "Get_array_values_fr_String.vi"("String Value"=w537) -> ("String array"=w536:string[])  [unwired: 1 out]
                  n282 = global write "Preference_global.vi" "LabVIEW Administrators"(w536) -> ()
                  n283 = local write "LabVIEW Administrators"(w536) -> ()
                }
                frame "SMTP server IP address" {
                  n284 = local write "SMTP server IP address"(w538) -> ()
                  n285 = global write "Preference_global.vi" "SMTP server IP address"(w538) -> ()
                }
                frame "Server Comms" {
                  n286 = Equal?(x="TRUE", y=w541) -> (x = y?=w540:bool)
                  n287 = case shown="False" w540 {
                    tunnel: [Server_Comms."Do Not Link To Server" ("Server Comms") Server_Comms."Server Link Healthy" ("Server Comms")] -> w539
                    frame False {
                    }
                    frame True {
                    }
                  }
                  n288 = local write "Server Comms"(w539) -> ()
                  n289 = global write "Preference_global.vi" "Server Comms"(w539) -> ()
                }
                frame "Temperature" {
                  n290 = global write "Preference_global.vi" "Temperature"(w545) -> ()
                  n291 = local write "Temperature"(w545) -> ()
                }
                frame "Abs Press (mbar)" {
                  n292 = global write "Preference_global.vi" "Abs Press (mbar)"(w546) -> ()
                  n293 = local write "Abs Press (mbar)"(w546) -> ()
                }
                frame "Qnet Site Root" {
                  n294 = String To Path(string=w548) -> (path=w547:path)
                  n295 = global write "Qnet_Globals.vi" "Local Site Root"(w547) -> ()
                  n296 = local write "Qnet Site Root"(w547) -> ()
                }
                frame "Current Overhead Factor" {
                  n297 = Fract/Exp String To Number(string=w550) -> (number=w549:dbl)  [unwired: 4 out]
                  n298 = call "Overhead_Factor.vi"("Current Overhead Factor In"=w549, "Mode"=Overhead."Initialise totals to 3hr") -> ()  [unwired: 2 in, 1 out]
                }
                frame "Auto Calib Error fr Previous" {
                  n299 = Fract/Exp String To Number(string=w553) -> (number=w552:dbl)  [unwired: 4 out]
                  n300 = global write "Preference_global.vi" "% Error From Previous Calib"(w552) -> ()
                  n301 = local write "% Error From Previous Calib"(w552) -> ()
                }
                frame "Auto Calib Error fr First" {
                  n302 = Fract/Exp String To Number(string=w555) -> (number=w554:dbl)  [unwired: 4 out]
                  n303 = global write "Preference_global.vi" "% Error From First Calib"(w554) -> ()
                  n304 = local write "% Error From First Calib"(w554) -> ()
                }
              }
            }
            frame "Char not in string" {
            }
          }
        }
        n305 = local read "Post Processing Machine"() -> (w509:bool)
        n306 = Select(t="Check file permission status", s=w509, f="is traverse setup blank?") -> (s? t:f=w507:string)
        n307 = Build Array (concatenate)(w511, w503) -> (w510:path[])
      }
      frame "is traverse setup blank?" {
        n308 = local read "Data Folder"() -> (w562:path)
        n309 = global read "Trav_pos_global.vi" "Default Traverse Setup"() -> (w556:string)
        n310 = Build Path(base path=w562, name or relative path="Preferences") -> (appended path=w561:path)
        n311 = Build Path(base path=w561, name or relative path=w565) -> (appended path=w560:path)
        n312 = List Folder(path=w560) -> (folder names=w558:string[])  [unwired: 1 in, 5 out]
        n313 = Search 1D Array(1D array=w558, element=w556) -> (index of element=w559:i32)  [unwired: 1 out]
        n314 = case shown="0, Default" w559 {
          tunnel: w558 -> [_ w571]
          tunnel: [w569 w570] -> w557
          tunnel: w556 -> [w569 _]
          frame 0, Default {
          }
          frame -1 {
            n315 = Index Array(array=w571, index=0) -> (element=w570:string)
          }
        }
        n316 = global write "Trav_pos_global.vi" "Default Traverse Setup"(w557) -> ()
      }
      frame "Please Enter new  Traverse Setup" {
        n317 = global read "Trav_pos_global.vi" "Default Traverse Setup"() -> (w575:string)
        n318 = String Length(string=w575) -> (length=w580:i32)
        n319 = In Range and Coerce(upper limit=w577, x=w580, lower limit=w578) -> (In Range?=w576:bool)  [unwired: 1 out]
        n320 = case shown="False" w576 {
          tunnel: w575 -> [w591 w599]
          tunnel: ["Please Enter new  Traverse Setup" "Update Traverse setup menu ring"] -> w579
          tunnel: [w584 w599] -> w574
          tunnel: w578 -> [w588 _]
          tunnel: w577 -> [w587 _]
          frame False {
            n321 = Format Into String(format string="Please Enter a Traverse Setup Name\nIt must be between %d and %d Characters" ("Message to user"), w588, w587) -> (resulting string=w586:string)  [unwired: 2 in, 1 out]
            n322 = call "Input_String_Dialog.vi"("Value"=w591, "Message to user"=w586) -> ("Ok Out"=w583:bool, "Output string"=w585:string)
            n323 = case shown="False" w583 {
              tunnel: w585 -> [_ w596]
              tunnel: [w592 w595] -> w584
              frame False {
                n324 = property on="Default Traverse Name" class="Ring (strict)"() -> ("Strings []"=w593:string[])  [unwired: 2 in, 2 out]
                n325 = Index Array(array=w593, index=0) -> (element=w592:string)
              }
              frame True {
                n326 = call "Fast_string_Replace.vi"("Replace match with:"="_", "Input String"=w596, "regular expression"=" ") -> ("Output String"=w595:string)  [unwired: 2 out]
              }
            }
          }
          frame True {
          }
        }
        n327 = global write "Trav_pos_global.vi" "Default Traverse Setup"(w574) -> ()
      }
      frame "Update Traverse setup menu ring" {
        n328 = global read "Trav_pos_global.vi" "Default Traverse Setup"() -> (w604:string)
        n329 = local read "Data Folder"() -> (w610:path)
        n330 = Build Path(base path=w610, name or relative path="Preferences") -> (appended path=w609:path)
        n331 = Build Path(base path=w609, name or relative path=w602) -> (appended path=w608:path)
        n332 = List Folder(path=w608) -> (folder names=w606:string[])  [unwired: 1 in, 5 out]
        n333 = Build Array (concatenate)(w606, "--New Traverse Setup--") -> (w605:string[])
        n334 = Search 1D Array(1D array=w605, element=w604) -> (index of element=w612:i32)  [unwired: 1 out]
        n335 = case shown="-1" w612 {
          tunnel: [w618 0] -> w614
          tunnel: w605 -> [w617 w621]
          tunnel: w604 -> [_ w620]
          tunnel: w612 -> [w618 _]
          tunnel: [w617 w619] -> w603
          frame 0, Default {
          }
          frame -1 {
            n336 = Build Array (concatenate)(w620, w621) -> (w619:string[])
          }
        }
        n337 = local write "Default Traverse Name"(w614) -> ()
        n338 = property on="Default Traverse Name" class="Ring (strict)"("Strings []"=w603) -> ()  [unwired: 2 in, 2 out]
      }
      frame "Create Traverse setup" {
        n339 = local read "Templates"() -> (w624:path)
        n340 = Build Path(base path=w624, name or relative path="All_Traverses") -> (appended path=w630:path)
        n341 = stacked-sequence {
          seq-local: [w635 _] -> [_ w663]
          seq-local: [w634 _] -> [_ _]
          tunnel: w630 -> [w637 _]
          tunnel: [w640 _] -> w627
          tunnel: [w639 _] -> w626
          tunnel: w624 -> [_ w662]
          tunnel: [_ w660] -> w623
          frame #0 {
            w643 = "Default_Space_file.xls" ("name or relative path")
            w638 = "Traverse_Setup.xls" ("name or relative path")
            n342 = global read "Trav_pos_global.vi" "Default Traverse Setup"() -> (w634:string)
            n343 = global read "Constants_global.vi" "Traverse folder"() -> (w647:path)
            n344 = Build Path(base path=w637, name or relative path=w643) -> (appended path=w641:path)
            n345 = Build Path(base path=w637, name or relative path=w638) -> (appended path=w636:path)
            n346 = Build Path(base path=w647, name or relative path=w634) -> (appended path=w635:path)
            n347 = Build Path(base path=w635, name or relative path="Trav_Space_Files") -> (appended path=w644:path)
            n348 = Build Path(base path=w644, name or relative path=w643) -> (appended path=w640:path)
            n349 = call "Does_file_exist_(simple).vi"("Pathname"=w640) -> ("exists?"=w642:bool)
            n350 = case shown="False" w642 {
              tunnel: w641 -> [w650 _]
              tunnel: w640 -> [w649 _]
              frame False {
                n351 = call "Create_directory_path.vi"("Path name"=w649) -> ("Path name Out"=w648:path)
                n352 = Copy(10:w648, 11:w650) -> ()  [unwired: 1 in, 5 out]
              }
              frame True {
              }
            }
            n353 = Build Path(base path=w635, name or relative path=w638) -> (appended path=w639:path)
            n354 = call "Does_file_exist_(simple).vi"("Pathname"=w639) -> ("exists?"=w646:bool)
            n355 = case shown="False" w646 {
              tunnel: w636 -> [w659 _]
              tunnel: w639 -> [w655 _]
              tunnel: w634 -> [w658 _]
              frame False {
                w651 = TRUE  # append to file? (new file:F)
                n356 = call "Create_directory_path.vi"("Path name"=w655) -> ("Path name Out"=w654:path)
                n357 = call "Read_File_Simple.vi"("Filename"=w659) -> ("string"=w657:string)  [unwired: 2 in, 7 out]
                n358 = call "Fast_string_Replace.vi"("Replace match with:"=w658, "Input String"=w657, "regular expression"="A_Tunnel") -> ("Output String"=w653:string)  [unwired: 2 out]
                n359 = call "Write_Characters_To_File.vi"("file path (dialog if empty)"=w654, "advisory dialog? (display:T)"=TRUE, "character string"=w653, "append to file? (new file:F)"=w651) -> ()  [unwired: 1 in, 4 out]
              }
              frame True {
              }
            }
          }
          frame #1 {
            w661 = "Traverse_Preferences.txt" ("name or relative path")
            n360 = Build Path(base path=w663, name or relative path=w661) -> (appended path=w660:path)
            n361 = Build Path(base path=w662, name or relative path=w661) -> (appended path=w664:path)
            n362 = call "Does_file_exist_(simple).vi"("Pathname"=w660) -> ("exists?"=w665:bool)
            n363 = case shown="False" w665 {
              tunnel: w664 -> [w668 _]
              tunnel: w660 -> [w667 _]
              frame False {
                n364 = call "Create_directory_path.vi"("Path name"=w667) -> ("Path name Out"=w666:path)
                n365 = Copy(10:w666, 11:w668) -> ()  [unwired: 1 in, 5 out]
              }
              frame True {
              }
            }
          }
        }
        n366 = Build Array (concatenate)(w629, w626, w623, w627) -> (w628:path[])
      }
      frame "Check file permission status" {
        n367 = for {
          tunnel: w673 -> [w687] mode=indexing
          shift-right: [w684] -> w670
          shift-left: "" -> [w685]
          n368 = call "Can_File_be_Editted.vi"("Filename"=w687) -> ("File Permissions OK?"=w688:bool, "Comment String"=w686:string)  [unwired: 2 out]
          n369 = case shown="False" w688 {
            tunnel: w687 -> [w693 _]
            tunnel: w686 -> [w692 _]
            tunnel: w685 -> [w691 w694]
            tunnel: [w690 w694] -> w684
            frame False {
              n370 = Format Into String(format string="\"%s\" %s\n", initial string=w691, w693, w692) -> (resulting string=w690:string)  [unwired: 1 in, 1 out]
            }
            frame True {
            }
          }
        }
        n371 = case shown="\"Load, Edit then Save\"" w674 {
          tunnel: ["Output Dev Number" w696 "Output Dev Number"] -> w675
          frame "Save Preferences to file" {
          }
          frame "Load, Edit then Save" {
            n372 = local read "Post Processing Machine"() -> (w699:bool)
            n373 = Select(t="Data Folder Changed?", s=w699, f="What next1") -> (s? t:f=w696:string)
          }
          frame "Load Preferences from file" {
          }
        }
        n374 = Empty String/Path?(string/path=w670) -> (empty?=w671:bool)
        n375 = case shown="True" w671 {
          tunnel: w670 -> [w683 _]
          frame False {
            n376 = Concatenate Strings("The following file permissions need to be sorted out before the software will run correctly.\n\n" ("string"), w683) -> (w681:string)
            n377 = Two Button Dialog(message=w681, 1:"Continue" ("F button name (\"Cancel\")"), 2:"Abort" ("F button name (\"Cancel\")")) -> (T button?=w678:bool)
            n378 = Stop(stop? (T)=w678) -> ()
          }
          frame True {
          }
        }
      }
      frame "What next1" {
        n379 = property on="Rig Setup" class="Ring (strict)"() -> ("Strings []"=w703:string[])  [unwired: 2 in, 2 out]
        n380 = Array Size(array=w703) -> (size(s)=w707:i32)
        n381 = Decrement(x=w707) -> (x-1=w706:i32)
        n382 = Equal?(x=w706, y="Rig Setup") -> (x = y?=w705:bool)
        n383 = case shown="False" w705 {
          tunnel: [w711 "Please Enter New Rig Name" ("t")] -> w704
          tunnel: w703 -> [w714 _]
          tunnel: "Rig Setup" -> [w713 _]
          frame False {
            n384 = global read "Preference_global.vi" "Rig Setup"() -> (w715:string)
            n385 = Index Array(array=w714, index=w713) -> (element=w710:string)
            n386 = Not Equal?(x=w710, y=w715) -> (x != y?=w712:bool)
            n387 = case shown="False" w712 {
              tunnel: ["What next2" ("f") "Update Rig setup menu ring" ("t")] -> w711
              tunnel: w710 -> [_ w717]
              frame False {
              }
              frame True {
                n388 = global write "Preference_global.vi" "Rig Setup"(w717) -> ()
              }
            }
          }
          frame True {
            n389 = global write "Preference_global.vi" "Rig Setup"("") -> ()
          }
        }
      }
      frame "What next2" {
        n390 = property on="Default Traverse Name" class="Ring (strict)"() -> ("Strings []"=w723:string[])  [unwired: 2 in, 2 out]
        n391 = Array Size(array=w723) -> (size(s)=w727:i32)
        n392 = Decrement(x=w727) -> (x-1=w726:i32)
        n393 = Equal?(x=w726, y="Default Traverse Name") -> (x = y?=w725:bool)
        n394 = case shown="False" w725 {
          tunnel: [w731 "Please Enter new  Traverse Setup" ("t")] -> w724
          tunnel: w723 -> [w735 _]
          tunnel: "Default Traverse Name" -> [w734 _]
          frame False {
            n395 = global read "Trav_pos_global.vi" "Default Traverse Setup"() -> (w733:string)
            n396 = Index Array(array=w735, index=w734) -> (element=w730:string)
            n397 = Not Equal?(x=w730, y=w733) -> (x != y?=w732:bool)
            n398 = case shown="False" w732 {
              tunnel: ["Data Folder Changed?" ("f") "Update Traverse setup menu ring" ("t")] -> w731
              tunnel: w730 -> [_ w737]
              frame False {
              }
              frame True {
                n399 = global write "Trav_pos_global.vi" "Default Traverse Setup"(w737) -> ()
              }
            }
          }
          frame True {
            n400 = global write "Trav_pos_global.vi" "Default Traverse Setup"("") -> ()
          }
        }
      }
      frame "Data Folder Changed?" {
        w742 = "Please Select your data folder"
        n401 = global read "Constants_global.vi" "Data Folder"() -> (w749:path)
        n402 = local read "Data Folder"() -> (w750:path)
        n403 = property on="OK" class="Bool (strict)"("Visible"=TRUE) -> ()  [unwired: 2 in, 2 out]
        n404 = while {
          shift-right: [w759] -> _
          shift-left: _ -> [w758]
          tunnel: [w757] -> w744
          stop <- TRUE stop-if-true
          n405 = local read "Post Processing Machine"() -> (w759:bool)
          n406 = Not Equal?(x=w759, y=w758) -> (x != y?=w757:bool)
        }
        n407 = Not Equal?(x=w749, y=w750) -> (x != y?=w748:bool)
        n408 = Select(t=w742, s=w748, f="Has OK has been pressed?") -> (s? t:f=w741:string)
        n409 = case shown="True" w744 {
          tunnel: [w753 w755] -> w743
          tunnel: w742 -> [_ w755]
          tunnel: w741 -> [w753 _]
          frame False {
          }
          frame True {
            n410 = global write "Preference_global.vi" "Rig Setup"("") -> ()
          }
        }
      }
      frame "Has OK has been pressed?" {
        n411 = flat-sequence {
          tunnel: ["OK"] -> w761
          frame #0 {
            n412 = Wait (ms)(milliseconds to wait=u32 100) -> ()  [unwired: 1 out]
          }
          frame #1 {
          }
        }
        n413 = local read "Post Processing Machine"() -> (w762:bool)
        n414 = case shown="False" w761 {
          tunnel: w762 -> [w767 w773]
          tunnel: [w766 w770] -> w760
          frame False {
            n415 = Select(t="Data Folder Changed?", s=w767, f="What next1") -> (s? t:f=w766:string)
          }
          frame True {
            n416 = Select(t="Save Preference File", s=w773, f="Output Dev Number") -> (s? t:f=w770:string)
          }
        }
      }
      frame "Output Dev Number" {
        n417 = stacked-sequence {
          seq-local: [w781 _ _] -> [_ w817 _]
          tunnel: w778 -> [_ _ _]
          frame #0 {
            w784 = T9 0 items=["Canonical Names Only"=0, "Aliases Only"=1, "Include Matching Aliases"=2, "Include All Aliases"=4] ("Search Mode")
            n418 = VISA Find Resource(10:w784) -> (3:w783:string[])  [unwired: 1 in, 3 out]
            n419 = for {
              shift-right: [w799] -> w781
              shift-left: string[] [] -> [w800]
              tunnel: w783 -> [w789] mode=indexing
              n420 = Reverse String(1:w789) -> (0:w797:string)
              n421 = Match Pattern(string=w797, regular expression="::") -> (before substring=w796:string)  [unwired: 4 out]
              n422 = Match Pattern(string=w789, regular expression="NI-VISA") -> (offset past match=w788:i32)  [unwired: 4 out]
              n423 = Reverse String(1:w796) -> (0:w794:string)
              n424 = Less Than 0?(x=w788) -> (x < 0?=w786:bool)
              n425 = Equal?(x=w794, y="INSTR") -> (x = y?=w792:bool)
              n426 = Equal?(x=w794, y="RAW") -> (x = y?=w791:bool)
              n427 = Or(x=w792, y=w791) -> (x .or. y?=w787:bool)
              n428 = And(x=w787, y=w786) -> (x .and. y?=w785:bool)
              n429 = case shown="True" w785 {
                tunnel: w800 -> [w801 w804]
                tunnel: [w801 w803] -> w799
                tunnel: w789 -> [_ w802]
                frame False {
                }
                frame True {
                  n430 = Build Array (concatenate)(w804, w802) -> (w803:string[])
                }
              }
            }
          }
          frame #1 {
            w809 = "Dev" ("format string")
            n431 = local read "Analogue Device Serial No."() -> (w813:string)
            n432 = String Length(string=w809) -> (length=w811:i32)
            n433 = local read "PWA Device Serial No."() -> (w807:string)
            n434 = String Subset(string=w813, length (rest)=w811) -> (substring=w815:string)  [unwired: 1 out]
            n435 = String Subset(string=w807, length (rest)=w811) -> (substring=w810:string)  [unwired: 1 out]
            n436 = Equal?(x=w815, y=w809) -> (x = y?=w812:bool)
            n437 = Equal?(x=w809, y=w810) -> (x = y?=w808:bool)
            n438 = for {
              tunnel: w813 -> [w836]
              tunnel: w817 -> [w834] mode=indexing
              tunnel: [w835] -> w829 mode=indexing
              tunnel: w807 -> [w833]
              tunnel: [w832] -> w826 mode=indexing
              n439 = Match Pattern(string=w834, regular expression=w836) -> (offset past match=w835:i32)  [unwired: 1 in, 3 out]
              n440 = Match Pattern(string=w834, regular expression=w833) -> (offset past match=w832:i32)  [unwired: 1 in, 3 out]
            }
            n441 = Array Max & Min(array=w829) -> (max index (indices)=w830:i32)  [unwired: 3 out]
            n442 = Array Max & Min(array=w826) -> (max index (indices)=w828:i32)  [unwired: 3 out]
            n443 = Increment(x=w828) -> (x+1=w819:i32)
            n444 = Increment(x=w830) -> (x+1=w823:i32)
            n445 = Equal To 0?(x=w823) -> (x = 0?=w825:bool)
            n446 = Equal To 0?(x=w819) -> (x = 0?=w820:bool)
            n447 = Select(t=1, s=w825, f=w823) -> (s? t:f=w824:i32)
            n448 = Select(t=1, s=w820, f=w819) -> (s? t:f=w818:i32)
            n449 = Format Into String(format string="Dev%d", w824) -> (resulting string=w814:string)  [unwired: 2 in, 1 out]
            n450 = Format Into String(format string="Dev%d", w818) -> (resulting string=w806:string)  [unwired: 2 in, 1 out]
            n451 = Select(t=w813, s=w812, f=w814) -> (s? t:f=w816:string)
            n452 = Select(t=w807, s=w808, f=w806) -> (s? t:f=w805:string)
            n453 = global write "PWAtasksGLOBAL.vi" "Analogue Dev Name"(w816) -> ()
            n454 = global write "PWAtasksGLOBAL.vi" "PWA Dev Name"(w805) -> ()
          }
          frame #2 {
            n455 = for {
              tunnel: string[] ["Raw_Calibrations", "Raw_Measurements", "Results", "Calibrations", "Commands"] -> [w841] mode=indexing
              n456 = call "Data_folder_Path.vi"("Data Type"=w841) -> ("Data Folder"=w840:path)  [unwired: 1 in]
              n457 = Build Path(base path=w840, name or relative path="Test" ("Substring")) -> (appended path=w843:path)
              n458 = call "Create_directory_path.vi"("Path name"=w843) -> ()  [unwired: 1 out]
            }
            n459 = call "Data_folder_Path.vi"("Data Type"="Results_Post_Processed" ("element")) -> ("Data Folder"=w837:path)  [unwired: 1 in]
            n460 = call "Create_directory_path.vi"("Path name"=w837) -> ()  [unwired: 1 out]
          }
        }
      }
      frame "Save Preference File" {
        n461 = call "Date_and_Time_to_string.vi"() -> ("Date and time (spreadsheet)"=w855:string)
        n462 = call "Setup_Filepath.vi"("Setup File Type"=Setup_Filetype."General", "Filename in"=w845) -> ("Filename Out"=w844:path)  [unwired: 1 out]
        n463 = for {
          tunnel: w854 -> [w865] mode=indexing
          shift-right: [w861] -> w853
          shift-left: w855 -> [w863]
          n464 = case shown="\"Analogue Device Serial No.\"" w865 {
            tunnel: w865 -> [w868 _ _ _ _ _ _ _ _ _ _ _ _ _ _ _ _]
            tunnel: ["No Match" "Server address" w871 w873 w875 w879 "SMTP server IP address" "PWA Device Serial No." "Analogue Device Serial No." w883 w885 "Temperature" "Abs Press (mbar)" w890 w895 w898 w901] -> w864
            frame "No Match", Default {
              n465 = call "Was_string_matched.vi"("Match Error"=TRUE, "Variable name"=w868) -> ()  [unwired: 1 in]
            }
            frame "Server address" {
              n466 = global write "Preference_global.vi" "Server address"("Server address") -> ()
            }
            frame "Server port number" {
              n467 = global write "Preference_global.vi" "Server port number"("Server port number") -> ()
              n468 = Number To Decimal String(number="Server port number") -> (decimal integer string=w871:string)  [unwired: 1 out]
            }
            frame "Default Source Establishment Time (s)" {
              n469 = global write "Preference_global.vi" "Default Source Establishment Time (s)"("Default Source Establishment Time (s)") -> ()
              n470 = Number To Decimal String(number="Default Source Establishment Time (s)") -> (decimal integer string=w873:string)  [unwired: 1 out]
            }
            frame "Tunnel Speed Control" {
              n471 = global write "Preference_global.vi" "Tunnel Speed Control"("Tunnel Speed Control") -> ()
              n472 = Select(t="TRUE", s="Tunnel Speed Control", f="FALSE") -> (s? t:f=w875:string)
            }
            frame "LabVIEW Administrators" {
              n473 = global write "Preference_global.vi" "LabVIEW Administrators"("LabVIEW Administrators") -> ()
              n474 = call "Put_Array_into_String.vi"("String array"="LabVIEW Administrators") -> ("String Value"=w879:string)
            }
            frame "SMTP server IP address" {
              n475 = global write "Preference_global.vi" "SMTP server IP address"("SMTP server IP address") -> ()
            }
            frame "PWA Device Serial No." {
            }
            frame "Analogue Device Serial No." {
            }
            frame "Default Traverse Name" {
              n476 = global read "Trav_pos_global.vi" "Default Traverse Setup"() -> (w883:string)
            }
            frame "Server Comms" {
              n477 = case shown="\"Server Link Healthy\"" "Server Comms" {
                tunnel: ["TRUE" "FALSE"] -> w885
                frame "Server Link Healthy" {
                }
                frame "Do Not Link To Server" {
                }
              }
              n478 = global write "Preference_global.vi" "Server Comms"("Server Comms") -> ()
            }
            frame "Temperature" {
              n479 = global write "Preference_global.vi" "Temperature"("Temperature") -> ()
            }
            frame "Abs Press (mbar)" {
              n480 = global write "Preference_global.vi" "Abs Press (mbar)"("Abs Press (mbar)") -> ()
            }
            frame "Current Overhead Factor" {
              n481 = call "Overhead_Factor.vi"("Mode"=Overhead."Read Current Overhead") -> ("Current Overhead Factor"=w892:dbl)  [unwired: 3 in]
              n482 = Number To Fractional String(number=w892, precision (6)=i16 4) -> (F-format string=w890:string)  [unwired: 2 out]
            }
            frame "Auto Calib Error fr Previous" {
              n483 = global write "Preference_global.vi" "% Error From Previous Calib"("% Error From Previous Calib") -> ()
              n484 = Number To Fractional String(number="% Error From Previous Calib", precision (6)=i16 2) -> (F-format string=w895:string)  [unwired: 2 out]
            }
            frame "Auto Calib Error fr First" {
              n485 = global write "Preference_global.vi" "% Error From First Calib"("% Error From First Calib") -> ()
              n486 = Number To Fractional String(number="% Error From First Calib", precision (6)=i16 2) -> (F-format string=w898:string)  [unwired: 2 out]
            }
            frame "Qnet Site Root" {
              n487 = global write "Qnet_Globals.vi" "Local Site Root"("Qnet Site Root") -> ()
              n488 = Path To String(path="Qnet Site Root") -> (string=w901:string)
            }
          }
          n489 = call "Characters_to_string.vi"("Characters to write"=w864, "Label for characters"=w865) -> ("Output string"=w862:string)
          n490 = Concatenate Strings(w863, w862) -> (w861:string)
        }
        n491 = case shown="\"Load, Edit then Save\"" w849 {
          tunnel: [TRUE TRUE TRUE] -> w848
          frame "Load, Edit then Save" {
            n492 = Current VI's Path() -> (path=w857:path)
            n493 = call "Open_Close_Front_Panel.ph.vi"("Front Panel Window:Open"=FALSE, "VI path"=w857) -> ()  [unwired: 2 out]
          }
          frame "Load Preferences from file" {
          }
          frame "Save Preferences to file" {
          }
        }
        n494 = call "Write_Characters_To_File.vi"("file path (dialog if empty)"=w844, "advisory dialog? (display:T)"=FALSE, "character string"=w853, "append to file? (new file:F)"=FALSE) -> ()  [unwired: 1 in, 4 out]
      }
      frame "Save SW Preferences" {
        w917 = FALSE  # append to file? (new file:F)
        w918 = FALSE  # advisory dialog? (display:T)
        n495 = local read "Post Processing Machine"() -> (w907:bool)
        n496 = Path To String(path="Data Folder") -> (string=w909:string)
        n497 = global read "Preference_global.vi" "Server Comms"() -> (w913:T2)
        n498 = call "Characters_to_string.vi"("Characters to write"=w909, "Label for characters"=w911) -> ("Output string"=w919:string)
        n499 = Select(t="True", s=w907, f="False") -> (s? t:f=w904:string)
        n500 = call "Characters_to_string.vi"("Characters to write"=w904, "Label for characters"=w902) -> ("Output string"=w903:string)
        n501 = call "Date_and_Time_to_string.vi"() -> ("Date and time (spreadsheet)"=w914:string)
        n502 = case shown="\"Server Link Healthy\"" w913 {
          tunnel: ["Update Served VI file" "Update Local Adam Table"] -> w912
          frame "Server Link Healthy" {
          }
          frame "Do Not Link To Server" {
          }
        }
        n503 = Concatenate Strings(w914, w919, w903) -> (w915:string)
        n504 = local read "EnFlo SW Preferences"() -> (w916:path)
        n505 = call "Write_Characters_To_File.vi"("file path (dialog if empty)"=w916, "advisory dialog? (display:T)"=w918, "character string"=w915, "append to file? (new file:F)"=w917) -> ()  [unwired: 1 in, 4 out]
      }
      frame "Update Local Adam Table" {
        n506 = stacked-sequence {
          seq-local: [w933 _] -> [_ w947]
          tunnel: ["Update Served VI file" _] -> w925
          frame #0 {
            w933 = T10 {"Ch Name"="", "Type"=enum."4011", "Function"=enum."Analogue Input", "Ch State"=enum."On", "Calibration type"=enum."Raw", "A"=0.0, "B"=0.0, "C"=0.0, "D"=0.0, "Comments"="", "Address"={"Main"=0, "Ch."=0, "Sub"=0, "Port Name"=""}, "String"="", "Duty"=0} ("Ch Discription")
            n507 = global read "Preference_global.vi" "Abs Press (mbar)"() -> (w930:string)
            n508 = global read "Preference_global.vi" "Temperature"() -> (w931:string)
            n509 = Bundle By Name(cluster=w933, "Type"=Module_type_ADAM."Hold Value", "Calibration type"=Calib_type_ADAM."Raw", "A"=1.0) -> (w934:T10)
            n510 = Build Array(w931, w930) -> (w929:string[])
            n511 = for {
              tunnel: [w940] -> w932 mode=indexing
              tunnel: w934 -> [w939]
              tunnel: w929 -> [w938] mode=indexing
              n512 = Bundle By Name(cluster=w939, "Ch Name"=w938) -> (w940:T10)
            }
            n513 = call "Update_Ch_Discription_client.vi"("Channels to update In"=w932) -> ()  [unwired: 1 out]
          }
          frame #1 {
            n514 = global read "Preference_global.vi" "Rig Setup"() -> (w942:string)
            n515 = call "Get_Current_Scan_client.vi"() -> ("Ch Description Array"=w948:T10[])  [unwired: 1 in, 3 out]
            n516 = Match Pattern(string=w942, regular expression="-") -> (before substring=w941:string)  [unwired: 4 out]
            n517 = Format Into String(format string="%s Metadata:" ("Format String"), w941) -> (resulting string=w950:string)  [unwired: 2 in, 1 out]
            n518 = Initialize Array(w947, 0 ("dimension size")) -> (w945:T10[])
            n519 = for {
              shift-right: [w961] -> w944
              shift-left: w945 -> [w962]
              tunnel: w948 -> [w953] mode=indexing
              tunnel: w950 -> [w960]
              tunnel: "Metadata:" ("Format String") -> [w959]
              n520 = Unbundle By Name(w953) -> ("Ch Name"=w952:string)
              n521 = Match Pattern(string=w952, regular expression=w960) -> (offset past match=w957:i32)  [unwired: 4 out]
              n522 = Match Pattern(string=w952, regular expression=w959) -> (offset past match=w958:i32)  [unwired: 4 out]
              n523 = Greater Or Equal To 0?(x=w958) -> (x >= 0?=w955:bool)
              n524 = Less Than 0?(x=w957) -> (x < 0?=w956:bool)
              n525 = And(x=w956, y=w955) -> (x .and. y?=w954:bool)
              n526 = case shown="True" w954 {
                tunnel: w962 -> [w963 w968]
                tunnel: [w963 w967] -> w961
                tunnel: w953 -> [_ w966]
                frame False {
                }
                frame True {
                  n527 = Bundle By Name(cluster=w966, "Ch State"=Channel_State."Off") -> (w964:T10)
                  n528 = Build Array (concatenate)(w968, w964) -> (w967:T10[])
                }
              }
            }
            n529 = call "Update_Ch_Discription_client.vi"("Channels to update In"=w944) -> ()  [unwired: 1 out]
          }
        }
      }
      frame "Update Served VI file" {
        # "Template"
        # "Orig"
        n530 = call "Setup_Filepath.vi"("Setup File Type"=Setup_Filetype."General", "Filename in"=w970) -> ("Filename Out"=w969:path)  [unwired: 1 out]
        n531 = Build Array("Served:VI:Name", "Served:VI:Path", "Server:IP Number:& Port No") -> (w975:string[])
        n532 = stacked-sequence {
          seq-local: [w980 _ _ _] -> [_ _ w990 _]
          seq-local: [_ w987 _ _] -> [_ _ w991 _]
          seq-local: [_ _ w992 _] -> [_ _ _ w1017]
          tunnel: w975 -> [w982 w988 _ w1018]
          tunnel: w969 -> [w981 _ _ w1019]
          tunnel: w970 -> [_ w984 _ _]
          frame #0 {
            n533 = call "Read_Ch_data_file.vi"("Present Channels"=w982, "Output"=enum16{"All Ch data", "The last few rows"}."All Ch data", "Filename"=w981) -> ("Channel Values"=w980:string[][])  [unwired: 2 in, 4 out]
          }
          frame #1 {
            n534 = local read "Templates"() -> (w986:path)
            n535 = Build Path(base path=w986, name or relative path=w984) -> (appended path=w985:path)
            n536 = call "Read_Ch_data_file.vi"("Present Channels"=w988, "Output"=enum16{"All Ch data", "The last few rows"}."All Ch data", "Filename"=w985) -> ("Channel Values"=w987:string[][])  [unwired: 2 in, 4 out]
          }
          frame #2 {
            n537 = Index Array(array=w990, index (col)=0 ("Index")) -> (element=w995:string[])  [unwired: 1 in]
            n538 = To Upper Case(1:w991) -> (0:w993:string[][])
            n539 = To Upper Case(1:w995) -> (0:w994:string[])
            n540 = for {
              tunnel: w994 -> [w998]
              tunnel: w991 -> [w1003] mode=indexing
              tunnel: w993 -> [w997] mode=indexing
              tunnel: [w1000] -> w992 mode=indexing
              tunnel: w990 -> [w999]
              n541 = Index Array(array=w997, index=0 ("Index")) -> (element=w1001:string)
              n542 = Search 1D Array(1D array=w998, element=w1001) -> (index of element=w1002:i32)  [unwired: 1 out]
              n543 = case shown="0, Default" w1002 {
                tunnel: w1003 -> [w1012 w1013]
                tunnel: w1002 -> [w1009 _]
                tunnel: [w1005 w1013] -> w1000
                tunnel: w999 -> [w1010 _]
                frame 0, Default {
                  n544 = Index Array(array=w1010, index (row)=w1009, index (col)=2 ("Index")) -> (element=w1007:string)
                  n545 = Array Subset(array=w1012, length=2) -> (w1006:string[])  [unwired: 1 in]
                  n546 = Build Array (concatenate)(w1006, w1007) -> (w1005:string[])
                }
                frame -1 {
                }
              }
            }
          }
          frame #3 {
            w1014 = FALSE  # Append last row only
            w1015 = FALSE  # Lock File
            w1016 = FALSE  # exists?
            n547 = call "Write_Ch_data_file.vi"("Append last row only"=w1014, "Lock File"=w1015, "exists?"=w1016, "Channel Values"=w1017, "Channel names"=w1018, "Filename"=w1019) -> ()  [unwired: 2 in, 4 out]
          }
        }
      }
      frame "Initialise Globals" {
        w1024 = TRUE  # OK
        w1028 = FALSE  # append to file? (new file:F)
        w1027 = FALSE  # advisory dialog? (display:T)
        n548 = global read "Constants_global.vi" "ADAM setups folder"() -> (w1034:path)
        n549 = global read "Constants_global.vi" "All_Users"() -> (w1023:path)
        n550 = property on="ADAM Setup File" class="Ring (strict)"() -> ("Strings []"=w1029:string[])  [unwired: 2 in, 2 out]
        n551 = Build Path(base path=w1023, name or relative path="Current_Username") -> (appended path=w1021:path)
        n552 = Build Path(base path=w1034, name or relative path="Setup_Files") -> (appended path=w1032:path)
        n553 = global read "Preference_global.vi" "User_Name"() -> (w1020:string)
        n554 = Build Path(base path=w1032, name or relative path="Selected_Filename.txt" ("Substring")) -> (appended path=w1025:path)
        n555 = call "Get_users_email_addresses.vi"("OK"=w1024) -> ()  [unwired: 5 out]
        n556 = Index Array(array=w1029, index="ADAM Setup File") -> (element=w1026:string)
        n557 = call "Write_File_Simple.vi"("character string"=w1020, "file path"=w1021) -> ()  [unwired: 1 in, 2 out]
        n558 = global write "Dynamic_call_global.ph.vi" "Acquisition Interlock"(FALSE ("Acquisition Interlock")) -> ()
        n559 = call "Write_Characters_To_File.vi"("file path (dialog if empty)"=w1025, "advisory dialog? (display:T)"=w1027, "character string"=w1026, "append to file? (new file:F)"=w1028) -> ()  [unwired: 1 in, 4 out]
      }
    }
  }
  n560 = call "Get_IP_Number.vi"() -> ("IP Number"=→"This Machine's IP Number":string)
